vi "NEW数据采集传输系统.vi"() -> ()   [LabVIEW 2016, in "数据传输系统.lvlib"]
uses:
  <vilib>/Averna/Notify Icon/NotifyIcon.llb/BalloonIcon.ctl
  <vilib>/Utility/miscctls.llb/LVPointTypeDef.ctl
  <vilib>/Utility/config.llb/Read Key (String).vi
  <vilib>/Averna/Notify Icon/NotifyIcon.llb/GetSelectedItemEvent.vi
  <vilib>/Averna/Notify Icon/NotifyIcon.llb/SetVisible.vi
  <vilib>/Averna/Notify Icon/NotifyIcon.llb/SetMenuDefaultItem.vi
  <vilib>/Averna/Notify Icon/NotifyIcon.llb/SetTipText.vi
  <vilib>/Utility/config.llb/NI_LVConfig.lvlib
  data/FreeMem.dll
  <vilib>/Averna/Notify Icon/NotifyIcon.llb/NotifyIcon.lvclass
  <vilib>/ptbypt/NI_PtbyPt.lvlib
panel:
  in  "updateconfiguration":T1={"主机"="27.154.58.30", "用户"="update", "密码"="std23506", "远程路径"="数据传输系统\\平台数据传输系统.exe", "下载文件名"="平台数据传输系统.exe", "软件版本"=""}
  out "标题显示":string
  in  "更新":bool
  out "错误输出":errorcluster
  in  "停止输入":bool caption="停止 2"
  in  "系统编码选择框":string(combo)="地表水质量监测"
  in  "数据发送通道":enum16{"TCP", "VISA"}(ring)
  in  "baud rate":u32=9600 caption="波特率"
  in  "VISA resource name":refnum<visa-resource-name> caption="VISA资源名称"
  in  "实时数据发送时间间隔/min":i32=1
  in  "数据组合发送":bool
  in  "日志、参数发送":bool
  in  "2011发送":bool
  in  "判断数据反馈":bool
  in  "数据发送协议":enum16{"2005-212协议", "2017-212协议"}(ring)=enum."2017-212协议"
  in  "重发时间":T2(ring)
  in  "重发日期":T3(ring)
  in  "开机启动":bool
  in  "确定更改起始时间":bool
  in  "更改起始时间":bool
  in  "数据发送起始时间":timestamp format="%<%.3X\n%Y/%m/%d>T"
  in  "每周自动重发":bool=TRUE
  in  "确定":bool
  in  "返回":bool
  in  "PW":string
  in  "MN":string
  in  "PORT":string
  in  "IP":string
  in  "站点设备":string
  in  "站点名称":string
  out "设置超时时间/min":i32=1
  out "状态信息":T4={"1st Error to Convert "=63, "步骤 "=enum."发送数据", "元素"="实时数据", "TCP服务端掉线计数"=0, "TCP掉线时间节点"="2019/05/08 15:24:17"} {"1st Error to Convert" items=["无错误", "参数错误", "内存已满", "超出区域", "文件结束", "文件已打开", "一般文件IO错误", "未找到文件", "文件权限错误", "磁盘已满", "路径副本", "打开过多文件", "未启用", "未找到资源文件", "无法添加资源", "未找到资源", "未找到图像", "图像内存错误", "画笔不存在", "配置错误类型", "配置未找到解析段", "配置解析错误", "配置内存错误", "错误外部代码格式", "错误外部代码偏移量", "外部代码不存在", "空窗口", "销毁窗口错误", "空菜单", "打印已中止", "错误打印记录", "打印驱动程序错误", "打印时窗口错误", "打印时内存错误", "打印对话框错误", "一般打印错误", "无效设备引用句柄", "设备未找到", "设备参数错误", "设备单位错误", "无法打开设备", "设备调用已中止", "一般错误", "用户已取消", "对象ID过低", "对象ID过高", "对象不在堆中", "未知的堆", "错误DefProc ID", "DefProc不在表格中", "范围外信息", "空方法", "未知信息", "不支持管理器调用", "错误地址", "连接过程中", "连接超时", "连接过程中", "不支持网络属性", "网络错误", "正在使用的地址", "系统缺少内存", "连接已中止", "连接已拒绝", "连接未建立", "连接已建立", "连接已关闭", "初始化错误（交互应用程序管理器）", "错误事件发生", "等待无约束事件发生处理程序", "事件发生队列溢出", "错误路径", "未发出信号量", "未识别类型（交互应用程序管理器）"]}
  out "数据接收超时指示灯":bool
  out "空闲时间/s":string
  out "系统时间":string
  out "实时小时数据上传":bool
  out "系统状态改变":bool
  out "软件版本":string
  out "掉线指示":bool
  out "核查数据上传":bool
  out "配置信息":T5
  in  "参数配置":bool
  out "反控数据发送":bool
  out "读取报文显示":string
  out "发送报文显示":string
  out "心跳包":bool
  out "通信状态":bool
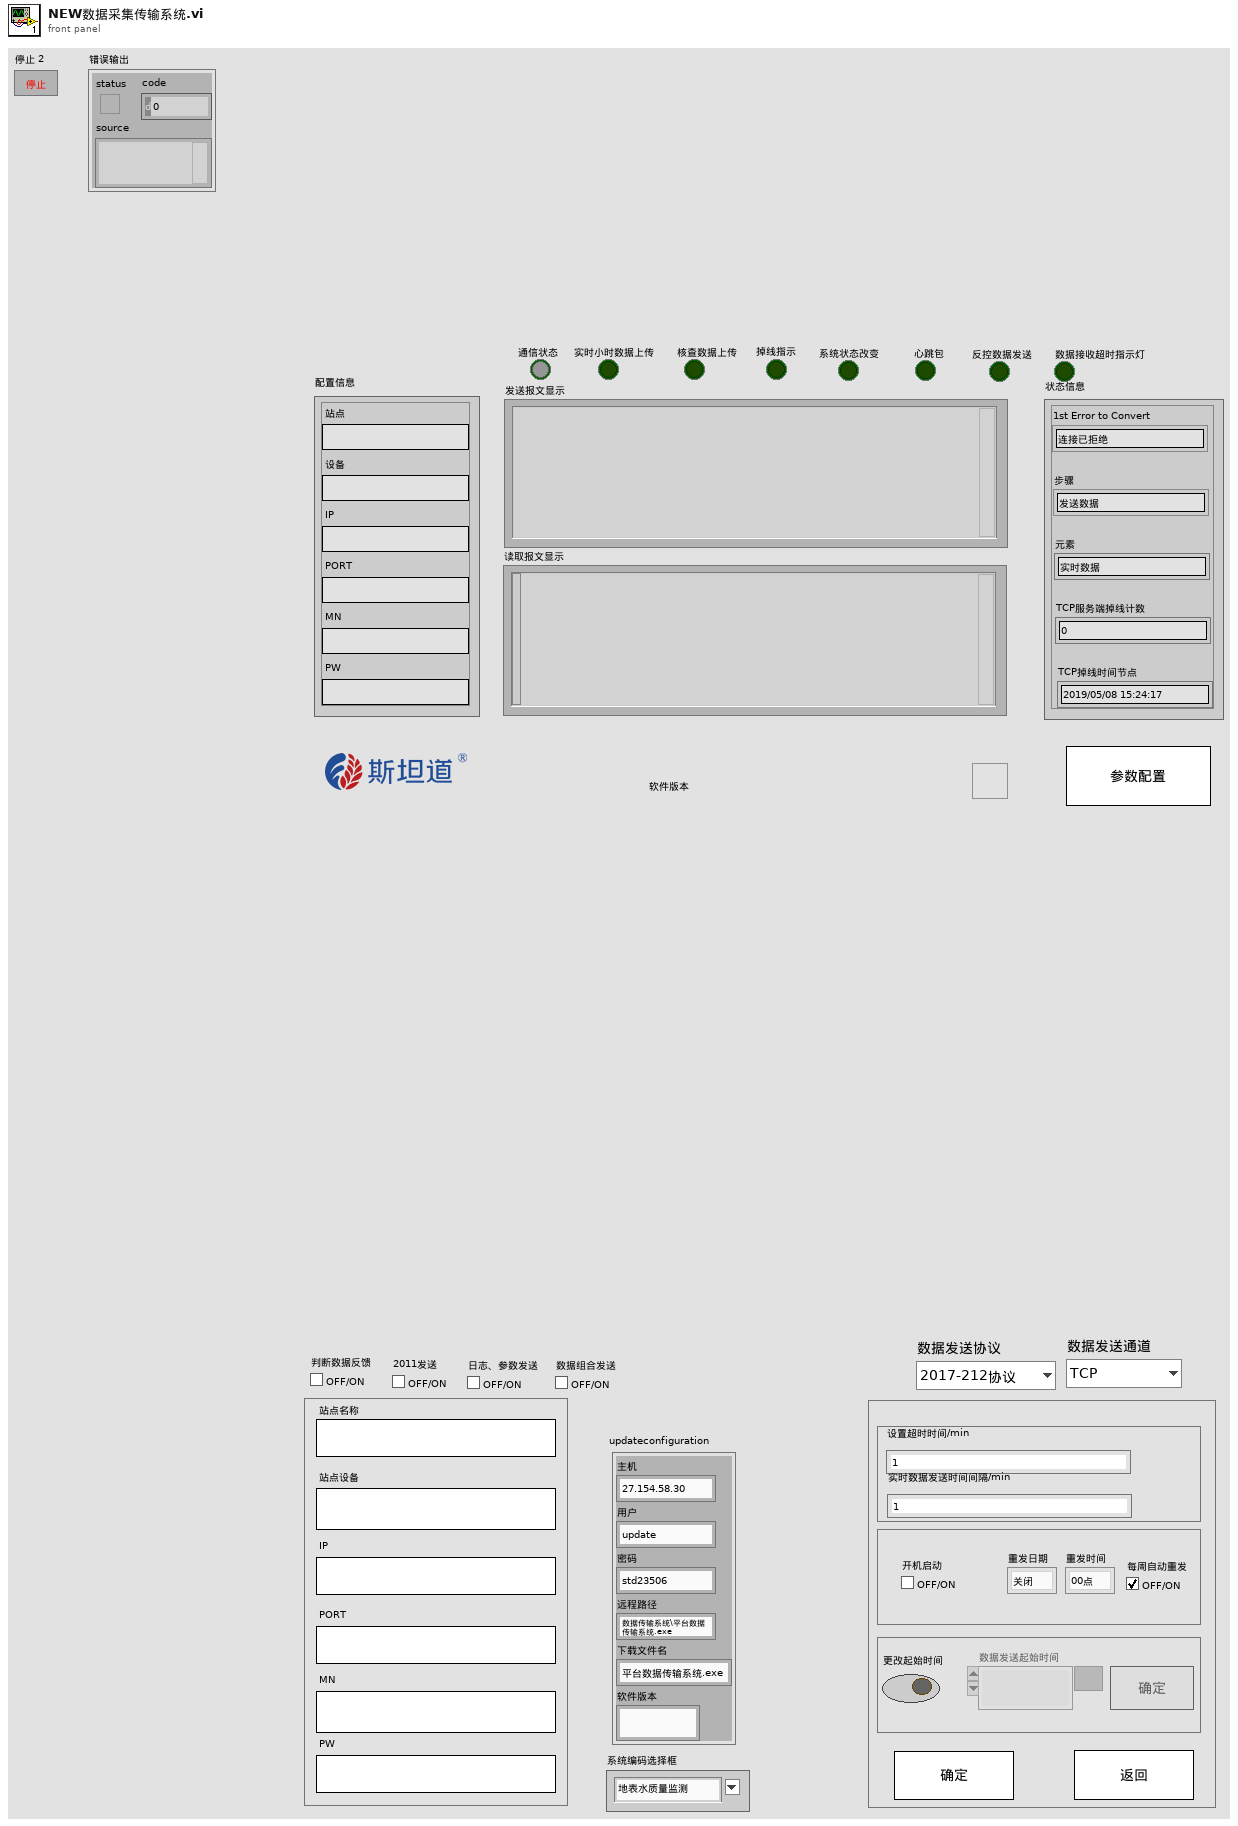
[diagram p1: front panel]
types:
  T1 = cluster{"主机":string, "用户":string, "密码":string, "远程路径":string, "下载文件名":string, "软件版本":string}
  T2 = enum16{"00点", "01点", "02点", "03点", "04点", "05点", "06点", "07点", "08点", "09点", "10点", "11点", "12点", "13点", "14点", "15点", "16点", "17点", "18点", "19点", "20点", "21点", "22点", "23点"}
  T3 = enum16{"关闭", "星期日", "星期一", "星期二", "星期三", "星期四", "星期五", "星期六"}
  T4 = cluster{"1st Error to Convert ":i32, "步骤 ":enum16{"打开连接", "发送数据", "读取数据", "数据处理", "关闭连接"}, "元素":string, "TCP服务端掉线计数":i32, "TCP掉线时间节点":string}
  T5 = cluster{"站点":string, "设备":string, "IP":string, "PORT":string, "MN":string, "PW":string}
  T6 = typedef "LVDateTimeRec.ctl" = cluster{"秒数的小数部分":dbl, "秒":i32, "分":i32, "时":i32, "日":i32, "月":i32, "年":i32, "天数（周）":i32, "天数（年）":i32, "DST":i32}
  T7 = enum32{"invalid app kind", "Development System", "Run Time System", "Student Edition", "Embedded LabVIEW", "Evaluation", "Custom"}
  T8 = typedef "LVPointTypeDef.ctl" = cluster{"Horizontal":i16, "Vertical":i16}
  T9 = cluster{"CODMn":bool, "CODCr":bool, "DO":bool, "铜":bool, "PH":bool, "氨氮":bool, "比电导率":bool, "水温":bool, "COD":bool, "浊度":bool, "总氮":bool, "总磷":bool, "叶绿素a":bool, "藻密度":bool, "水位":bool, "流速":bool, "瞬时流量":bool, "累积流量":bool, "亚硝酸盐":bool, "硫化物":bool, "ORP":bool, "铅":bool, "镉":bool, "锌":bool, "镍":bool, "锰":bool, "汞":bool}
  T10 = typedef "NI_LVConfig.lvlib/Config Data RefNum.ctl" = refnum<k1>
  T11 = typedef "imagedata.ctl" = cluster{"image type":i32, "image depth":i32, "image":u8[], "mask":u8[], "colors":u32[], "Rectangle":cluster{"left":i16, "top":i16, "right":i16, "bottom":i16}}
  T12 = cluster{"[0]":string, "[1]":string, "[2]":string, "[3]":string, "[4]":string, "[5]":string, "[6]":string, "[7]":string, "[8]":string, "[9]":string, "[10]":string, "[11]":string, "[12]":string, "[13]":string, "[14]":string, "[15]":string, "[16]":string, "[17]":string, "[18]":string, "[19]":string, "[20]":string, "[21]":string, "[22]":string, "[23]":string, "[24]":string, "[25]":string, "[26]":string}
  T13 = enum8{"Enabled", "Disabled", "Disabled and Grayed Out"}
  T14 = cluster{"[0]":string, "[1]":string, "[2]":string, "[3]":string, "[4]":string, "[5]":string, "[6]":string, "[7]":string}
  T15 = cluster{"[0]":string, "[1]":string, "[2]":string, "[3]":string, "[4]":string, "[5]":string, "[6]":string, "[7]":string, "[8]":string, "[9]":string, "[10]":string, "[11]":string, "[12]":string, "[13]":string, "[14]":string}
  T16 = enum32{"Invalid", "Standard", "Closed", "Hidden", "Minimized", "Maximized"}
  T17 = typedef "NotifyIcon.lvlib/NotifyIcon.lvclass/BalloonIcon.ctl" = enum32{"None", "Information", "Warning", "Error"}
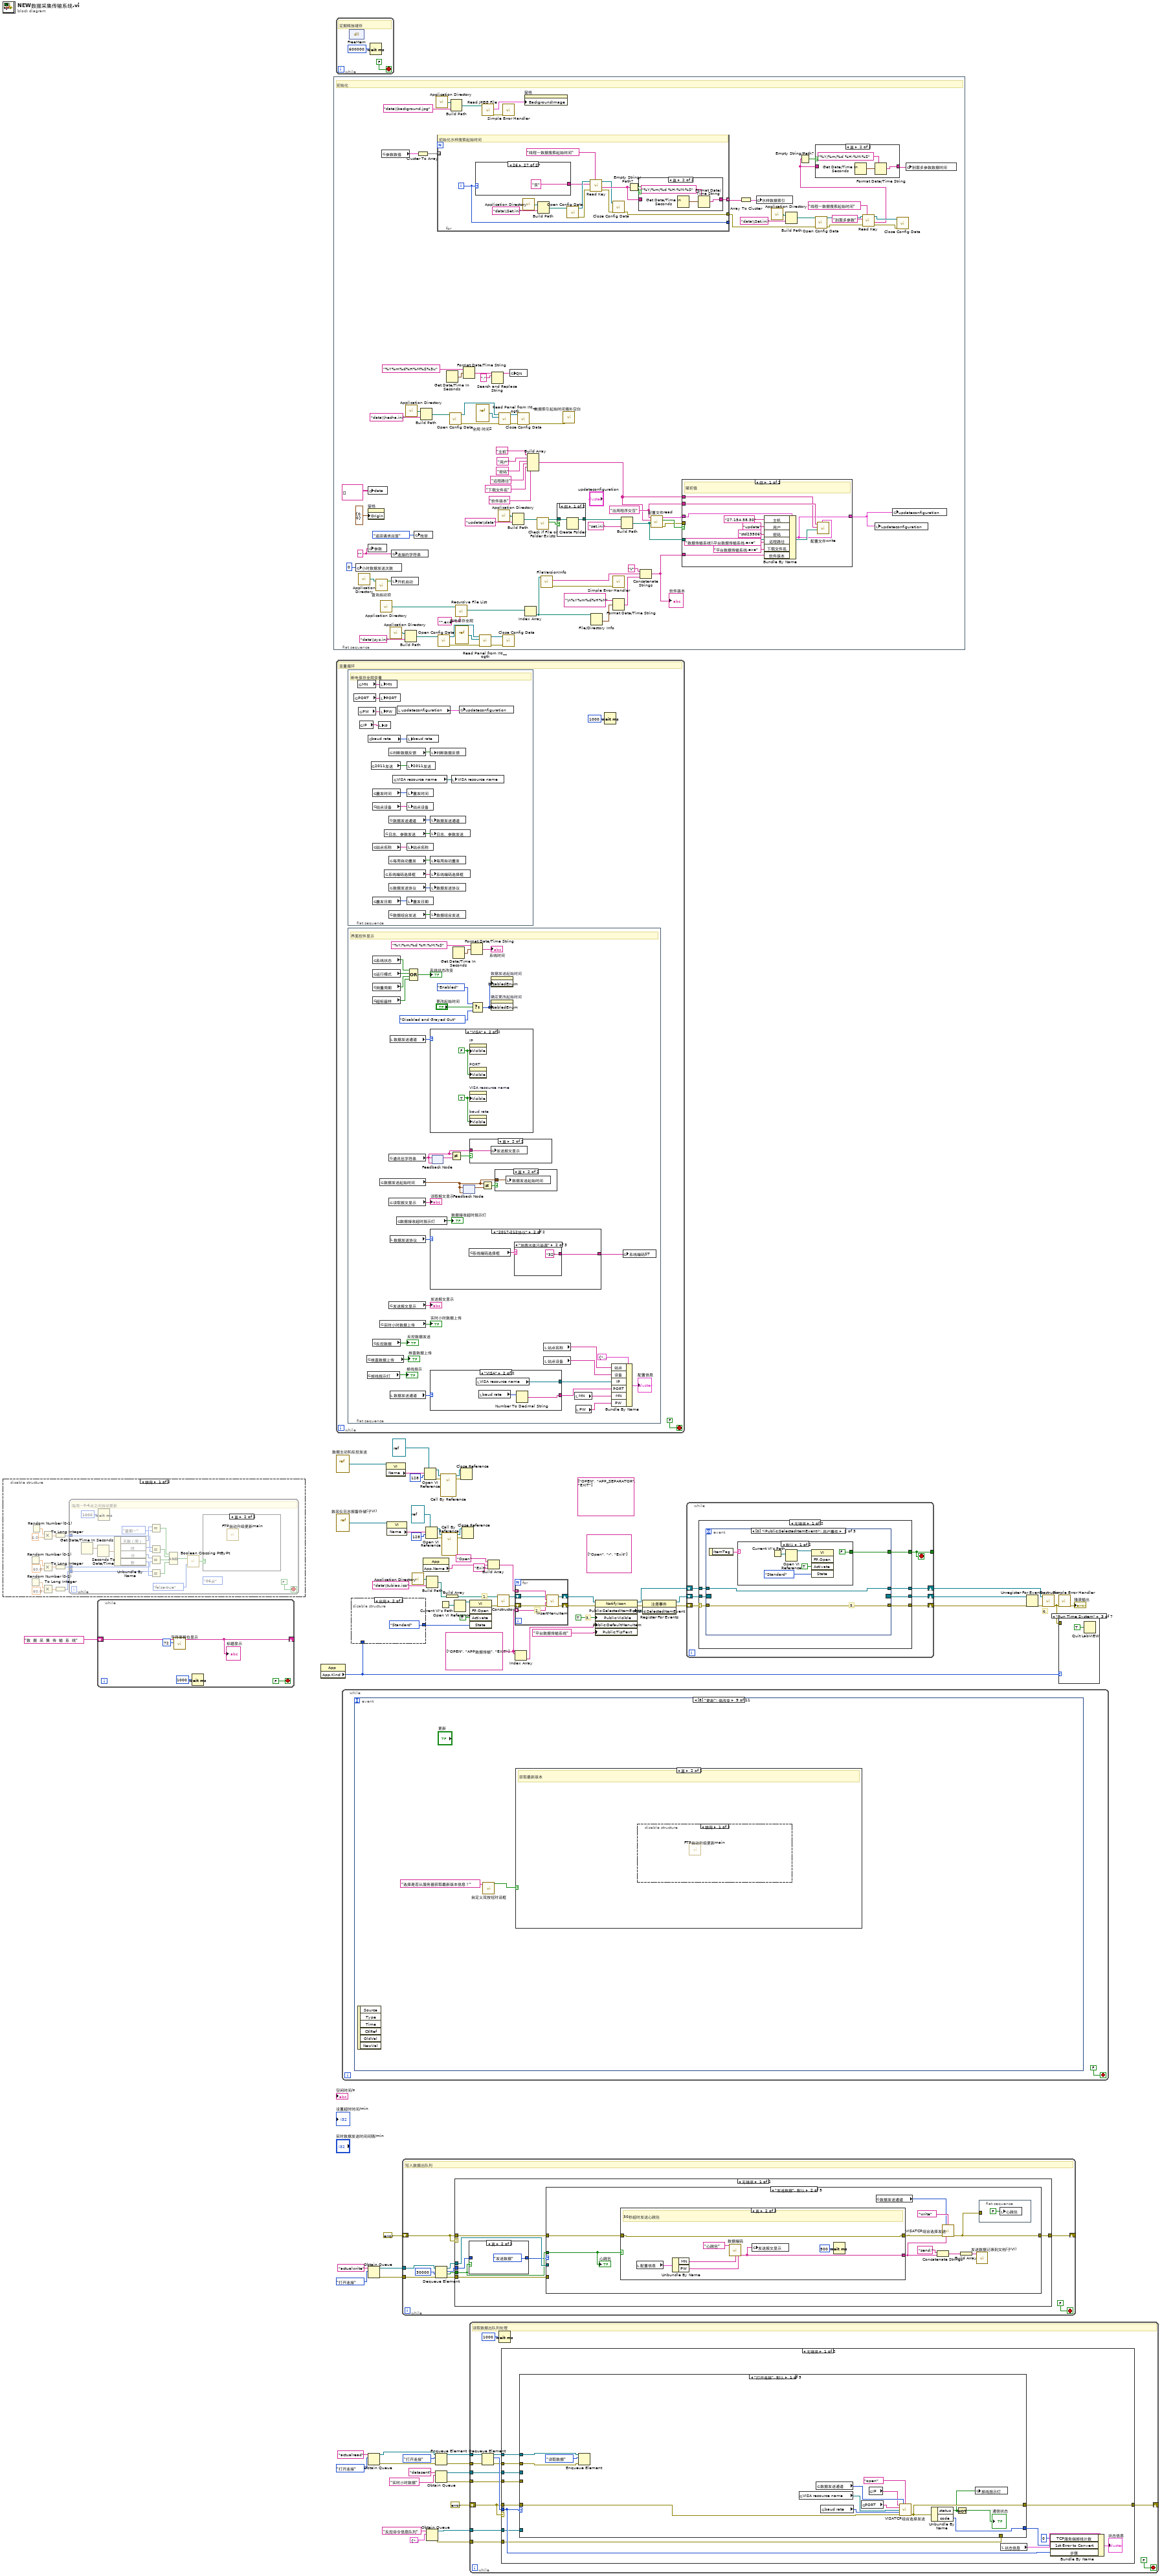
[diagram p0: block diagram]
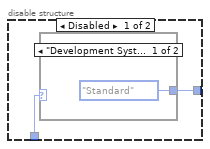
[diagram p4: hidden frame]
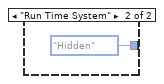
[diagram p5: hidden frame]
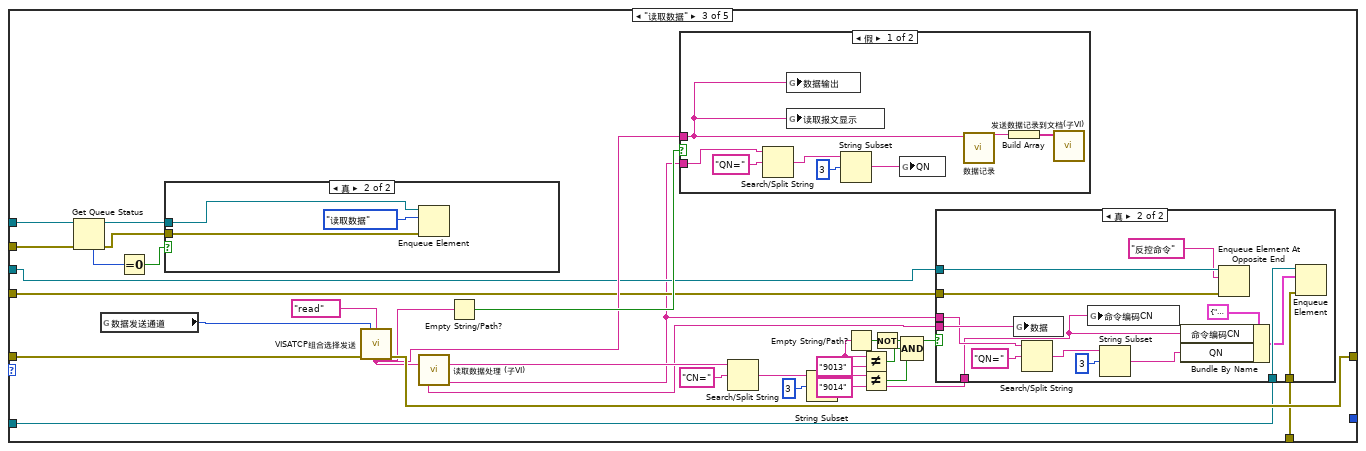
[diagram p7: hidden frame]
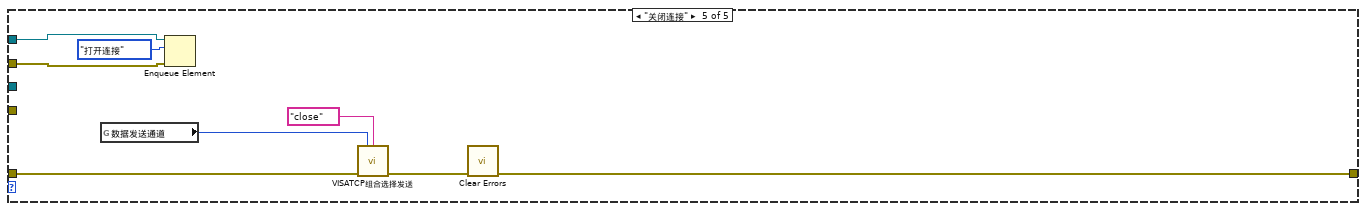
[diagram p12: hidden frame]
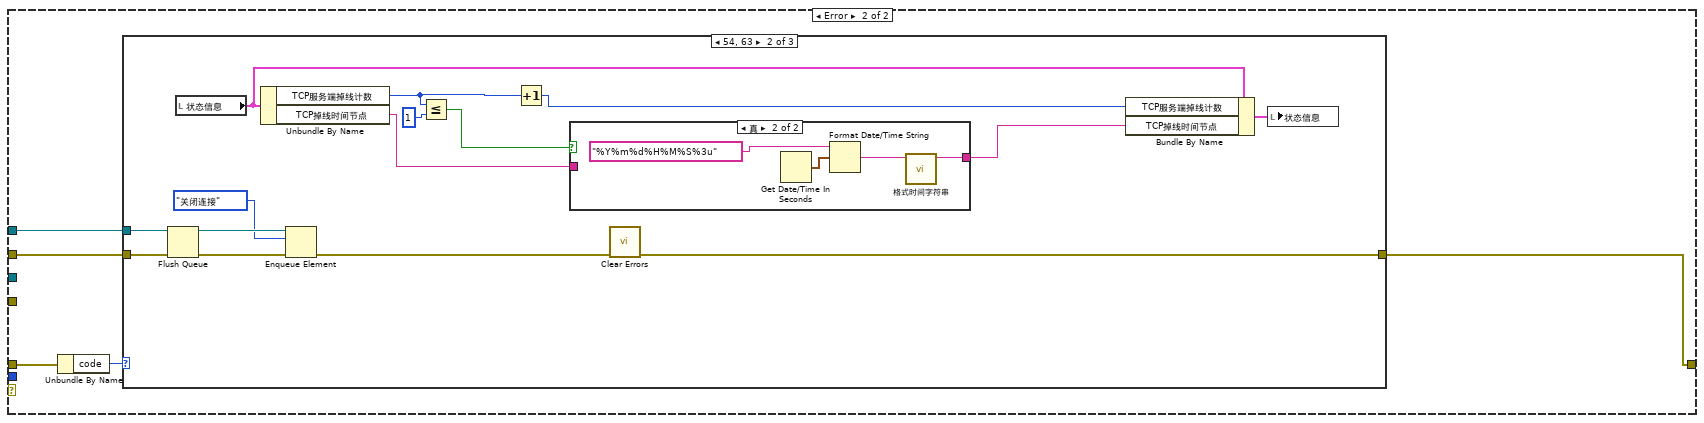
[diagram p13: hidden frame]
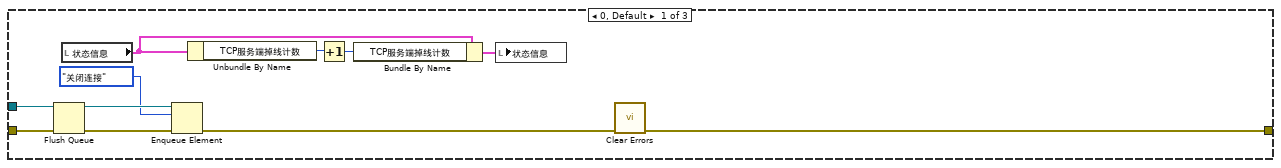
[diagram p14: hidden frame]
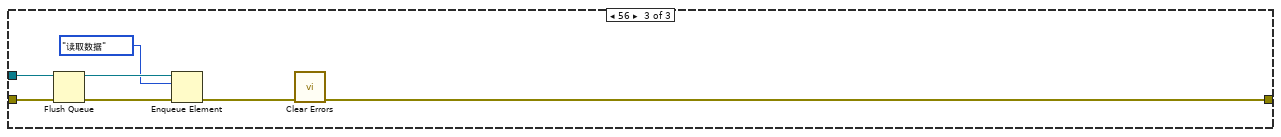
[diagram p16: hidden frame]
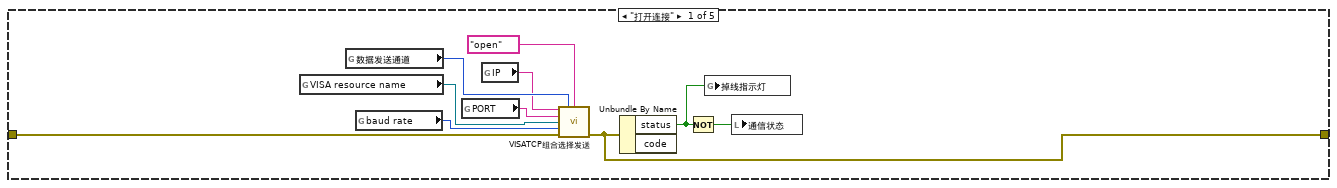
[diagram p18: hidden frame]
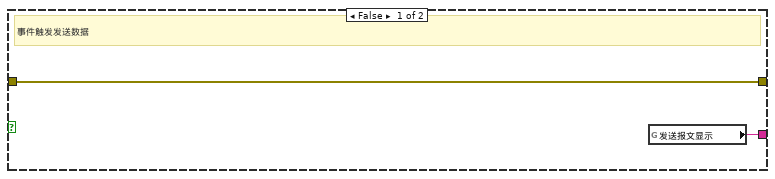
[diagram p19: hidden frame]
diagram:
  w1 = string[] ["OPEN", "APP数据传输", "EXIT"]
  (unwired) string[] ["OPEN", "APP_SEPARATOR", "EXIT"]
  (unwired) string[] ["Open", "-", "Exit"]
  # "6."
  # "3."
  # "1."
  n1 = disable-structure shown="禁用" {
    frame Disabled {
      n2 = Random Number (0-1)() -> (number: 0 to 1=w80:dbl)
      n3 = Random Number (0-1)() -> (number: 0 to 1=w79:dbl)
      n4 = Random Number (0-1)() -> (number: 0 to 1=w83:dbl)
      n5 = Multiply(x=w83, y=6.0) -> (x*y=w77:dbl)
      n6 = Multiply(x=w80, y=60.0) -> (x*y=w75:dbl)
      n7 = Multiply(x=w79, y=60.0) -> (x*y=w73:dbl)
      n8 = To Long Integer(number=w77) -> (32bit integer=w76:i32)
      n9 = To Long Integer(number=w75) -> (32bit integer=w74:i32)
      n10 = To Long Integer(number=w73) -> (32bit integer=w72:i32)
      n11 = while {
        tunnel: w76 -> [w91]
        tunnel: w74 -> [w86]
        tunnel: w72 -> [w85]
        stop <- FALSE stop-if-true
        (unwired) T2."06点" ("重发时间")
        # "每周一0-6点之间自动更新"
        n12 = Get Date/Time In Seconds() -> (seconds since 1Jan1904=w100:timestamp)
        n13 = Seconds To Date/Time(time stamp (now)=w100) -> (date time rec=w96:T6)  [unwired: 1 in]
        n14 = Wait (ms)(milliseconds to wait=u32 1000 ("等待时间（毫秒）")) -> ()  [unwired: 1 out]
        n15 = Unbundle By Name(w96) -> ("天数（周）"=w99:i32, "时"=w93:i32, "分"=w90:i32, "秒"=w88:i32)
        n16 = Equal?(x=w99, y=T3."星期一" ("重发日期")) -> (x = y?=w98:bool)
        n17 = Equal?(x=w93, y=w91) -> (x = y?=w97:bool)
        n18 = Equal?(x=w90, y=w86) -> (x = y?=w89:bool)
        n19 = Equal?(x=w85, y=w88) -> (x = y?=w87:bool)
        n20 = Compound Arithmetic op=AND ("复合运算")(w98, w97, w89, w87) -> (w95:bool)
        n21 = call <vilib>:"Boolean Crossing PtByPt.vi"("direction"=enum16{"either", "false-true", "true-false"}."false-true", "input"=w95) -> ("crossing"=w84:bool)  [unwired: 1 in]
        n22 = case shown="真" w84 {
          frame False {
          }
          frame True {
            n23 = call "FTP自动升级更新main.vi"() -> ()  [unwired: 12 in]
          }
        }
      }
    }
    frame Enabled {
    }
  }
  n24 = while {
    shift-right: [w104] -> _
    shift-left: "数  据  采  集  传  输  系  统" ("标题显示") -> [w105]
    stop <- FALSE stop-if-true
    n25 = call "字符串移位显示.vi"("字符框大小"=72, "字符串输入"=w105) -> ("移位后字符串"=w104:string)  [unwired: 8 in, 1 out]
    "标题显示" <- w104
    n26 = Wait (ms)(milliseconds to wait=u32 1000 ("等待时间（毫秒）")) -> ()  [unwired: 1 out]
  }
  n27 = property class="App"() -> ("App.Kind"=w46:T7)  [unwired: 2 in, 2 out]
  n28 = flat-sequence {
    frame #0 {
      w137 = "应用程序交互" ("section")
      w187 = "" ("参数")
      # "初始化"
      n29 = global write "全局 小时数据发送次数.vi" "小时数据发送次数"(0 ("数值")) -> ()
      n30 = call <vilib>:"Application Directory.vi"() -> ("Application Directory"=w157:path)
      n31 = global write "全局 实时数据参数.vi" "data"(string[][] [] ("data")) -> ()
      n32 = property on="窗格" class="Pane"("Origin"=T8 {"Horizontal"=0, "Vertical"=0} ("原点")) -> ()  [unwired: 2 in, 2 out]
      n33 = global write "全局 实时数据参数.vi" "参数"(w187) -> ()
      n34 = call "查询启动项.vi"("启动文件路径"=w157) -> ("包含启动项"=w156:bool)  [unwired: 9 in, 1 out]
      n35 = call <vilib>:"Application Directory.vi"() -> ("Application Directory"=w167:path)
      n36 = global read "全局1.vi" "参数数值"() -> (w143:T9)
      n37 = call <vilib>:"Application Directory.vi"() -> ("Application Directory"=w161:path)
      n38 = global write "全局 实时数据参数.vi" "连接的字符串"(w187) -> ()
      n39 = local write "开机启动"(w156) -> ()
      n40 = Build Path(base path=w161, name or relative path="data\\sys.ini" ("名称或相对路径")) -> (appended path=w159:path)
      n41 = call <vilib>:"Application Directory.vi"() -> ("Application Directory"=w151:path)
      n42 = global write "全局1.vi" "枚举"(enum16{"返回请求应答", "上传数据", "返回执行结果"}."返回请求应答" ("枚举")) -> ()
      n43 = Cluster To Array(cluster=w143) -> (array=w144:bool[])
      n44 = Build Path(base path=w151, name or relative path="data\\hecha.ini" ("名称或相对路径")) -> (appended path=w153:path)
      n45 = call <vilib>:"Application Directory.vi"() -> ("Application Directory"=w178:path)
      n46 = for {
        tunnel: w144 -> [_] mode=indexing
        tunnel: [w219] -> _
        tunnel: [w216] -> w142 mode=indexing
        tunnel: [w215] -> w117
        i -> [w219]
        # "初始化水样搜索起始时间"
        n47 = case shown="26" w219 {
          tunnel: ["CODMn" "CODCr" "DO" "铜" "PH" "氨氮" "比电导率" "水温" "COD" "浊度" "总氮" "总磷" "叶绿素a" "藻密度" "水位" "流速" "瞬时流量" "累积流量" "亚硝氮" "硫化物" "ORP" "铅" "镉" "锌" "镍" "锰" "汞"] -> w222
          frame 0, Default {
          }
          frame 1 {
          }
          frame 2 {
          }
          frame 3 {
          }
          frame 4 {
          }
          frame 5 {
          }
          frame 6 {
          }
          frame 7 {
          }
          frame 8 {
          }
          frame 9 {
          }
          frame 10 {
          }
          frame 11 {
          }
          frame 12 {
          }
          frame 13 {
          }
          frame 14 {
          }
          frame 15 {
          }
          frame 16 {
          }
          frame 17 {
          }
          frame 18 {
          }
          frame 19 {
          }
          frame 20 {
          }
          frame 21 {
          }
          frame 22 {
          }
          frame 23 {
          }
          frame 24 {
          }
          frame 25 {
          }
          frame 26 {
          }
        }
        n48 = call <vilib>:"Application Directory.vi"() -> ("Application Directory"=w228:path)
        n49 = Build Path(base path=w228, name or relative path="data\\Set.ini" ("名称或相对路径")) -> (appended path=w226:path)
        n50 = call <vilib>:"Open Config Data.vi"("configuration file path"=w226) -> ("error out"=w224:errorcluster, "refnum"=w225:T10)  [unwired: 8 in, 1 out]
        n51 = call-poly <vilib>:"Read Key.vi"("section"="线程一数据搜索起始时间", "error in (no error)"=w224, "key"=w222, "refnum"=w225) -> ("error out"=w217:errorcluster, "value"=w220:string, "refnum out"=w218:T10)  [unwired: 4 in, 1 out]
        n52 = call <vilib>:"Close Config Data.vi"("error in (no error)"=w217, "refnum"=w218) -> ("error out"=w215:errorcluster)  [unwired: 8 in, 1 out]
        n53 = Empty String/Path?(string/path=w220) -> (empty?=w221:bool)
        n54 = case shown="真" w221 {
          tunnel: [w229 w230] -> w216
          tunnel: w220 -> [w229 _]
          frame False {
          }
          frame True {
            n55 = Get Date/Time In Seconds() -> (seconds since 1Jan1904=w232:timestamp)
            n56 = Format Date/Time String(time format string (%c)="%Y/%m/%d %H:%M:%S" ("时间格式字符串(%c)"), seconds (now)=w232) -> (date/time string=w230:string)  [unwired: 1 in]
          }
        }
      }
      n57 = call <vilib>:"Open Config Data.vi"("configuration file path"=w159) -> ("error out"=w165:errorcluster, "refnum"=w164:T10)  [unwired: 8 in, 1 out]
      n58 = Get Date/Time In Seconds() -> (seconds since 1Jan1904=w183:timestamp)
      n59 = call <vilib>:"Open Config Data.vi"("configuration file path"=w153) -> ("error out"=w147:errorcluster, "refnum"=w148:T10)  [unwired: 8 in, 1 out]
      n60 = Build Path(base path=w178, name or relative path="data\\background.jpg" ("名称或相对路径")) -> (appended path=w177:path)
      n61 = call <vilib>:"Recursive File List.vi"("pattern"="*.exe", "Folder Path"=w167) -> ("All Files in Dir"=w173:path[])  [unwired: 5 in, 4 out]
      n62 = vi-ref "断电保存全局.vi"() -> (w163:refnum<vi>)
      n63 = Format Date/Time String(time format string (%c)="%Y%m%d%H%M%S%3u" ("时间格式字符串(%c)"), seconds (now)=w183) -> (date/time string=w182:string)  [unwired: 1 in]
      n64 = vi-ref "全局 时间2.vi"() -> (w149:refnum<vi>)
      n65 = call <userlib>:"Read Panel from INI__ogtk.vi"("error in (no error)"=w165, "VI ref"=w163, "refnum"=w164) -> ("error out"=w158:errorcluster, "refnum out"=w162:T10)  [unwired: 7 in]
      n66 = call <vilib>:"Read JPEG File.vi"("path to JPEG file"=w177) -> ("error out"=w175:errorcluster, "image data"=w176:T11)  [unwired: 8 in, 1 out]
      n67 = Search and Replace String(input string=w182, search string="." ("搜索字符串")) -> (result string=w180:string)  [unwired: 6 in, 3 out]
      n68 = call <vilib>:"Application Directory.vi"() -> ("Application Directory"=w123:path)
      n69 = call <userlib>:"Read Panel from INI__ogtk.vi"("error in (no error)"=w147, "VI ref"=w149, "refnum"=w148) -> ("error out"=w146:errorcluster, "refnum out"=w150:T10)  [unwired: 7 in]
      n70 = call <vilib>:"Simple Error Handler.vi"("error in (no error)"=w175) -> ()  [unwired: 4 in, 5 out]
      n71 = call <vilib>:"Close Config Data.vi"("error in (no error)"=w158, "refnum"=w162) -> ()  [unwired: 8 in, 2 out]
      n72 = global write "全局1.vi" "QN"(w180) -> ()
      n73 = Build Path(base path=w123, name or relative path="update\\data" ("名称或相对路径")) -> (appended path=w124:path)
      n74 = call <vilib>:"Close Config Data.vi"("error in (no error)"=w146, "refnum"=w150) -> ("error out"=w145:errorcluster)  [unwired: 8 in, 1 out]
      n75 = property on="窗格" class="Pane"("BackgroundImage"=w176) -> ()  [unwired: 2 in, 2 out]
      n76 = Index Array(array=w173) -> (element=w172:path)  [unwired: 1 in]
      n77 = Build Array("主机" ("section"), "用户" ("section"), "密码" ("key"), "远程路径" ("key"), "下载文件名" ("key"), "软件版本" ("key")) -> (w127:string[])
      n78 = call <vilib>:"Check if File or Folder Exists.vi"("path"=w124) -> ("file or folder exists?"=w125:bool, "dup path"=w126:path)  [unwired: 8 in, 1 out]
      n79 = call <vilib>:"FileVersionInfo.vi"("Application Path in"=w172) -> ("error out"=w166:errorcluster, "File Version Info"=w154:string)  [unwired: 7 in, 2 out]
      n80 = case shown="假" w125 {
        tunnel: w126 -> [w195 w196]
        tunnel: [w194 w196] -> w121
        frame False {
          n81 = Create Folder(path (use dialog)=w195) -> (created path=w194:path)  [unwired: 2 in, 2 out]
        }
        frame True {
        }
      }
      n82 = call "数据索引起始时间填补空白.vi"("error in (no error)"=w145) -> ()  [unwired: 10 in, 1 out]
      n83 = File/Directory Info(path=w172) -> (last mod=w171:timestamp)  [unwired: 1 in, 6 out]
      n84 = call <vilib>:"Simple Error Handler.vi"("error in (no error)"=w166) -> ()  [unwired: 4 in, 5 out]
      n85 = Format Date/Time String(time format string (%c)="\n%Y%m%d%H%M" ("时间格式字符串(%c)"), seconds (now)=w171) -> (date/time string=w168:string)  [unwired: 1 in]
      n86 = Build Path(base path=w121, name or relative path="set.ini" ("名称或相对路径")) -> (appended path=w136:path)
      n87 = Concatenate Strings("V" ("字符串"), w154, w168) -> (w138:string)
      "软件版本" <- w138
      n88 = call "配置文件read.vi"("configuration file path"=w136, "键数组"=w127, "段"=w137) -> ("error out"=w135:errorcluster, "section exists?"=w140:bool, "updateconfiguration"=w139:T1)  [unwired: 6 in]
      n89 = case shown="假" w140 {
        tunnel: w139 -> [w203 w209]
        tunnel: [w202 w208] -> w134
        tunnel: w138 -> [w197 w214]
        tunnel: w137 -> [w206 w213]
        tunnel: w127 -> [w205 w212]
        tunnel: w136 -> [w204 w211]
        tunnel: w135 -> [_ w210]
        frame False {
          # "赋初值"
          n90 = Bundle By Name(cluster=w203, "主机"="27.154.58.30" ("key"), "用户"="update", "密码"="std23506", "远程路径"="数据传输系统\\平台数据传输系统.exe", "下载文件名"="平台数据传输系统.exe", "软件版本"=w197) -> (w202:T1)
          n91 = call "配置文件write.vi"("updateconfiguration"=w202, "configuration file path"=w204, "键数组"=w205, "段"=w206) -> ()  [unwired: 7 in, 1 out]
        }
        frame True {
          # "本地"
          n92 = Bundle By Name(cluster=w209, "软件版本"=w214) -> (w208:T1)
          n93 = call "配置文件write.vi"("updateconfiguration"=w208, "error in (no error)"=w210, "configuration file path"=w211, "键数组"=w212, "段"=w213) -> ()  [unwired: 6 in, 1 out]
        }
      }
      n94 = Array To Cluster(array=w142) -> (cluster=w141:T12)
      n95 = global write "全局 水样时间.vi" "水样数据索引"(w141) -> ()
      n96 = call <vilib>:"Application Directory.vi"() -> ("Application Directory"=w120:path)
      n97 = Build Path(base path=w120, name or relative path="data\\Set.ini" ("名称或相对路径")) -> (appended path=w118:path)
      n98 = call <vilib>:"Open Config Data.vi"("error in (no error)"=w117, "configuration file path"=w118) -> ("error out"=w114:errorcluster, "refnum"=w115:T10)  [unwired: 7 in, 1 out]
      n99 = call-poly <vilib>:"Read Key.vi"("section"="线程一数据搜索起始时间", "error in (no error)"=w114, "key"="剖面多参数", "refnum"=w115) -> ("error out"=w111:errorcluster, "value"=w109:string, "refnum out"=w112:T10)  [unwired: 4 in, 1 out]
      n100 = Empty String/Path?(string/path=w109) -> (empty?=w108:bool)
      n101 = case shown="真" w108 {
        tunnel: [w190 w191] -> w110
        tunnel: w109 -> [w190 _]
        frame False {
        }
        frame True {
          n102 = Get Date/Time In Seconds() -> (seconds since 1Jan1904=w193:timestamp)
          n103 = Format Date/Time String(time format string (%c)="%Y/%m/%d %H:%M:%S" ("时间格式字符串(%c)"), seconds (now)=w193) -> (date/time string=w191:string)  [unwired: 1 in]
        }
      }
      n104 = local write "updateconfiguration"(w134) -> ()
      n105 = global write "update全局.vi" "updateconfiguration"(w134) -> ()
      n106 = call <vilib>:"Close Config Data.vi"("error in (no error)"=w111, "refnum"=w112) -> ()  [unwired: 8 in, 2 out]
      n107 = global write "全局 水样时间.vi" "剖面多参数数据时间"(w110) -> ()
    }
  }
  n108 = while {
    stop <- FALSE stop-if-true
    # "定期释放缓存"
    n109 = dll-call lib="PTH2fabs F\tgitkrakenCC;平台数采程序 - V2（微站认证版） - 整点触发dataFreeMem.dll" fn="FreeMem"() -> ()  [unwired: 4 in, 2 out]
    n110 = Wait (ms)(milliseconds to wait=u32 600000 ("等待时间（毫秒）")) -> ()  [unwired: 1 out]
  }
  n111 = while {
    stop <- FALSE stop-if-true
    # "变量循环"
    n112 = flat-sequence {
      frame #0 {
        # "断电保存全局变量"
        n113 = global read "断电保存全局.vi" "PORT"() -> (w333:string)
        n114 = global read "断电保存全局.vi" "MN"() -> (w332:string)
        n115 = global read "断电保存全局.vi" "PW"() -> (w331:string)
        n116 = global read "断电保存全局.vi" "IP"() -> (w334:string)
        n117 = global read "断电保存全局.vi" "baud rate"() -> (w329:u32)
        n118 = global read "断电保存全局.vi" "2011发送"() -> (w325:bool)
        n119 = global read "断电保存全局.vi" "重发时间"() -> (w319:T2)
        n120 = global read "断电保存全局.vi" "站点设备"() -> (w335:string)
        n121 = global read "断电保存全局.vi" "站点名称"() -> (w336:string)
        n122 = global read "断电保存全局.vi" "重发日期"() -> (w327:T3)
        n123 = local write "IP"(w334) -> ()
        n124 = local write "MN"(w332) -> ()
        n125 = local write "PORT"(w333) -> ()
        n126 = local write "PW"(w331) -> ()
        n127 = global read "断电保存全局.vi" "日志、参数发送"() -> (w324:bool)
        n128 = global read "断电保存全局.vi" "系统编码选择框"() -> (w320:string)
        n129 = global read "断电保存全局.vi" "判断数据反馈"() -> (w326:bool)
        n130 = global read "断电保存全局.vi" "数据发送通道"() -> (w321:enum16{"TCP", "VISA"})
        n131 = global read "断电保存全局.vi" "每周自动重发"() -> (w328:bool)
        n132 = global read "断电保存全局.vi" "数据发送协议"() -> (w322:enum16{"2005-212协议", "2017-212协议"})
        n133 = global read "断电保存全局.vi" "数据组合发送"() -> (w323:bool)
        n134 = global read "断电保存全局.vi" "VISA resource name"() -> (w330:refnum<visa-resource-name>)
        n135 = local read "updateconfiguration"() -> (w318:T1)
        n136 = local write "baud rate"(w329) -> ()
        n137 = local write "2011发送"(w325) -> ()
        n138 = local write "重发时间"(w319) -> ()
        n139 = local write "站点设备"(w335) -> ()
        n140 = local write "站点名称"(w336) -> ()
        n141 = local write "重发日期"(w327) -> ()
        n142 = local write "判断数据反馈"(w326) -> ()
        n143 = local write "数据发送通道"(w321) -> ()
        n144 = local write "日志、参数发送"(w324) -> ()
        n145 = local write "每周自动重发"(w328) -> ()
        n146 = local write "系统编码选择框"(w320) -> ()
        n147 = local write "数据发送协议"(w322) -> ()
        n148 = local write "数据组合发送"(w323) -> ()
        n149 = local write "VISA resource name"(w330) -> ()
        n150 = global write "update全局.vi" "updateconfiguration"(w318) -> ()
      }
    }
    n151 = flat-sequence {
      frame #0 {
        # "界面控件显示"
        n152 = global read "全局1.vi" "核查数据上传"() -> (→"核查数据上传":bool)
        n153 = global read "全局 数据发送重叠.vi" "掉线指示灯"() -> (→"掉线指示":bool)
        n154 = global read "全局1.vi" "系统状态"() -> (w267:bool)
        n155 = global read "全局1.vi" "运行模式"() -> (w268:bool)
        n156 = global read "全局1.vi" "测量周期"() -> (w269:bool)
        n157 = global read "全局1.vi" "超标留样"() -> (w270:bool)
        n158 = global read "全局1.vi" "反控数据"() -> (→"反控数据发送":bool)
        n159 = global read "全局1.vi" "数据发送起始时间"() -> (w264:timestamp)
        n160 = global read "全局1.vi" "实时小时数据上传"() -> (→"实时小时数据上传":bool)
        n161 = global read "全局1.vi" "通讯包字符串"() -> (w281:string)
        n162 = global read "全局1.vi" "读取报文显示"() -> (→"读取报文显示":string)
        n163 = global read "全局1.vi" "发送报文显示"() -> (→"发送报文显示":string)
        n164 = local read "数据发送通道"() -> (w275:enum16{"TCP", "VISA"})
        n165 = local read "数据发送协议"() -> (w289:enum16{"2005-212协议", "2017-212协议"})
        n166 = local read "数据发送通道"() -> (w300:enum16{"TCP", "VISA"})
        n167 = global read "全局 数据发送重叠.vi" "数据接收超时指示灯"() -> (→"数据接收超时指示灯":bool)
        n168 = Compound Arithmetic op=OR ("复合运算")(w267, w268, w269, w270) -> (→"系统状态改变":bool)
        n169 = case shown="\"VISA\"" w275 {
          frame "TCP", Default {
            w302 = TRUE ("可见")
            w303 = FALSE ("可见")
            n170 = property on="IP" class="Str"("Visible"=w302) -> ()  [unwired: 2 in, 2 out]
            n171 = property on="PORT" class="Str"("Visible"=w302) -> ()  [unwired: 2 in, 2 out]
            n172 = property on="VISA resource name" class="VISAName"("Visible"=w303) -> ()  [unwired: 2 in, 2 out]
            n173 = property on="baud rate" class="DigNum (严格)"("Visible"=w303) -> ()  [unwired: 2 in, 2 out]
          }
          frame "VISA" {
            w304 = FALSE ("可见")
            w305 = TRUE ("可见")
            n174 = property on="IP" class="Str"("Visible"=w304) -> ()  [unwired: 2 in, 2 out]
            n175 = property on="PORT" class="Str"("Visible"=w304) -> ()  [unwired: 2 in, 2 out]
            n176 = property on="VISA resource name" class="VISAName"("Visible"=w305) -> ()  [unwired: 2 in, 2 out]
            n177 = property on="baud rate" class="DigNum (严格)"("Visible"=w305) -> ()  [unwired: 2 in, 2 out]
          }
        }
        n178 = case shown="\"2017-212协议\"" w289 {
          tunnel: ["32" ("设备编码MN") w308] -> w288
          frame "2005-212协议", Default {
          }
          frame "2017-212协议" {
            n179 = global read "断电保存全局.vi" "系统编码选择框"() -> (w309:string)
            n180 = case shown="\"地表水体污染源\"" w309 {
              tunnel: ["52" ("设备编码MN") "32" ("设备编码MN") "21" ("设备编码MN")] -> w308
              frame "污水排放过程监测" {
              }
              frame "地表水体污染源" {
              }
              frame "地表水质量监测", Default {
              }
            }
          }
        }
        n181 = case shown="\"VISA\"" w300 {
          tunnel: [w314 w317] -> w297
          tunnel: [w313 w315] -> w294
          frame "TCP", Default {
            n182 = local read "PORT"() -> (w313:string)
            n183 = local read "IP"() -> (w314:string)
          }
          frame "VISA" {
            n184 = local read "VISA resource name"() -> (w317:refnum<visa-resource-name>)
            n185 = local read "baud rate"() -> (w316:u32)
            n186 = Number To Decimal String(number=w316) -> (decimal integer string=w315:string)  [unwired: 1 in]
          }
        }
        n187 = feedback #1(w281) -> (w282:string)
        n188 = feedback-in #1(w281) -> ()
        n189 = Not Equal?(x=w281, y=w282) -> (x != y?=w280:bool)
        n190 = Get Date/Time In Seconds() -> (seconds since 1Jan1904=w290:timestamp)
        n191 = feedback #2(w264) -> (w266:timestamp)
        n192 = feedback-in #2(w264) -> ()
        n193 = case shown="真" w280 {
          tunnel: w281 -> [_ w306]
          frame False {
          }
          frame True {
            n194 = global write "全局1.vi" "发送报文显示"(w306) -> ()
          }
        }
        n195 = Format Date/Time String(time format string (%c)="%Y/%m/%d %H:%M:%S" ("时间格式字符串(%c)"), seconds (now)=w290) -> (date/time string=→"系统时间":string)  [unwired: 1 in]
        n196 = Select(t=T13."Enabled" ("禁用"), s="更改起始时间", f=T13."Disabled and Grayed Out" ("禁用")) -> (s? t:f=w276:T13)
        n197 = Not Equal?(x=w264, y=w266) -> (x != y?=w265:bool)
        n198 = property on="数据发送起始时间" class="AbsTime (严格)"("DisabledEnum"=w276) -> ()  [unwired: 2 in, 2 out]
        n199 = property on="确定更改起始时间" class="Bool"("DisabledEnum"=w276) -> ()  [unwired: 2 in, 2 out]
        n200 = case shown="真" w265 {
          tunnel: w264 -> [_ w301]
          frame False {
          }
          frame True {
            n201 = local write "数据发送起始时间"(w301) -> ()
          }
        }
        n202 = local read "站点名称"() -> (w296:string)
        n203 = local read "站点设备"() -> (w295:string)
        n204 = local read "MN"() -> (w293:string)
        n205 = local read "PW"() -> (w292:string)
        n206 = Bundle By Name(cluster=T5 {"站点"="", "设备"="", "IP"="", "PORT"="", "MN"="", "PW"=""} ("配置信息"), "站点"=w296, "设备"=w295, "IP"=w297, "PORT"=w294, "MN"=w293, "PW"=w292) -> (→"配置信息":T5)
        n207 = global write "全局1.vi" "系统编码ST"(w288) -> ()
      }
    }
    n208 = Wait (ms)(milliseconds to wait=u32 1000 ("等待时间（毫秒）")) -> ()  [unwired: 1 out]
  }
  n209 = vi-ref "数据主动和反控发送.vi"() -> (w37:refnum<vi>)
  n210 = vi-ref "数采仪日志报警存储(子VI).vi"() -> (w38:refnum<vi>)
  n211 = while {
    stop <- FALSE stop-if-true
    n212 = event shown="[8] \"更新\": 值改变" {
      selector: _ -> [_ _ _ _ _ _ _ _ _ _ _]
      dyn-events: _ -> [_ _ _ _ _ _ _ _ _ _ _]
      timeout: _ -> [_ _ _ _ _ _ _ _ _ _ _]
      event Timeout {
        n213 = event-data() -> ()  [unwired: 1 in, 3 out]
      }
      event "站点名称", "站点设备", "IP", "PORT", "MN", "PW", "VISA resource name", "baud rate", "系统编码选择框", "每周自动重发", "重发日期", "重发时间": Value Change {
        n214 = event-data() -> ()  [unwired: 1 in, 6 out]
        n215 = flat-sequence {
          frame #0 {
            n216 = global write "断电保存全局.vi" "PW"("PW") -> ()
            n217 = global write "断电保存全局.vi" "站点名称"("站点名称") -> ()
            n218 = global write "断电保存全局.vi" "MN"("MN") -> ()
            n219 = global write "断电保存全局.vi" "PORT"("PORT") -> ()
            n220 = global write "断电保存全局.vi" "IP"("IP") -> ()
            n221 = global write "断电保存全局.vi" "重发日期"("重发日期") -> ()
            n222 = global write "断电保存全局.vi" "重发时间"("重发时间") -> ()
            n223 = global write "断电保存全局.vi" "站点设备"("站点设备") -> ()
            n224 = global write "断电保存全局.vi" "baud rate"("baud rate") -> ()
            n225 = global write "断电保存全局.vi" "系统编码选择框"("系统编码选择框") -> ()
            n226 = global write "断电保存全局.vi" "每周自动重发"("每周自动重发") -> ()
            n227 = global write "断电保存全局.vi" "VISA resource name"("VISA resource name") -> ()
          }
          frame #1 {
            n228 = call <vilib>:"Application Directory.vi"() -> ("Application Directory"=w350:path)
            n229 = Build Path(base path=w350, name or relative path="data\\sys.ini" ("名称或相对路径")) -> (appended path=w352:path)
            n230 = call <vilib>:"Open Config Data.vi"("configuration file path"=w352) -> ("error out"=w356:errorcluster, "refnum"=w353:T10)  [unwired: 8 in, 1 out]
            n231 = vi-ref "断电保存全局.vi"() -> (w354:refnum<vi>)
            n232 = call <userlib>:"Write Panel to INI__ogtk.vi"("error in (no error)"=w356, "VI ref"=w354, "refnum"=w353) -> ("error out"=w357:errorcluster, "refnum out"=w355:T10)  [unwired: 7 in]
            n233 = call <vilib>:"Close Config Data.vi"("error in (no error)"=w357, "refnum"=w355) -> ("error out"=w362:errorcluster, "file path"=w363:path)  [unwired: 8 in]
            n234 = Open/Create/Replace File(file path (use dialog)=w363, error in=w362) -> (refnum out=w359:refnum<file>, error out=w358:errorcluster)  [unwired: 4 in, 1 out]
            n235 = Flush File(refnum=w359, error in=w358) -> (refnum out=w360:refnum<file>, error out=w361:errorcluster)
            n236 = Close File(refnum=w360, error in=w361) -> ()  [unwired: 2 out]
          }
        }
      }
      event "数据发送通道", "数据发送协议", "数据组合发送", "2011发送", "日志、参数发送", "判断数据反馈": Value Change {
        n237 = event-data() -> ("CtlRef"=w367:refnum<vi>, "OldVal"=w365:variant, "NewVal"=w364:variant)  [unwired: 1 in, 3 out]
        n238 = property class="Ctl"(reference=w367) -> ("Label.Text"=w366:string)  [unwired: 1 in, 2 out]
        n239 = case shown="\"数据发送通道\"" w366 {
          tunnel: w365 -> [_ w371 w394 w417 w440 w463 w486]
          tunnel: w364 -> [_ w368 w391 w414 w437 w460 w483]
          frame "假", Default {
          }
          frame "数据发送通道" {
            n240 = Variant To Data(type=enum16{"TCP", "VISA"}."TCP" ("数据发送通道"), Variant=w368) -> (data=w369:enum16{"TCP", "VISA"})  [unwired: 1 in, 1 out]
            n241 = global write "断电保存全局.vi" "数据发送通道"(w369) -> ()
            n242 = Two Button Dialog(message="TCP通过网络发送数据，VISA通过串口发送数据，确定更改数据发送通道吗？" ("消息")) -> (T button?=w372:bool)  [unwired: 2 in]
            n243 = case shown="假" w372 {
              tunnel: w371 -> [w375 _]
              frame False {
                n244 = Variant To Data(type=enum16{"TCP", "VISA"}."TCP" ("数据发送通道"), Variant=w375) -> (data=w374:enum16{"TCP", "VISA"})  [unwired: 1 in, 1 out]
                n245 = global write "断电保存全局.vi" "数据发送通道"(w374) -> ()
              }
              frame True {
                n246 = flat-sequence {
                  frame #0 {
                  }
                  frame #1 {
                    n247 = call <vilib>:"Application Directory.vi"() -> ("Application Directory"=w377:path)
                    n248 = Build Path(base path=w377, name or relative path="data\\sys.ini" ("名称或相对路径")) -> (appended path=w379:path)
                    n249 = call <vilib>:"Open Config Data.vi"("configuration file path"=w379) -> ("error out"=w383:errorcluster, "refnum"=w380:T10)  [unwired: 8 in, 1 out]
                    n250 = vi-ref "断电保存全局.vi"() -> (w381:refnum<vi>)
                    n251 = call <userlib>:"Write Panel to INI__ogtk.vi"("error in (no error)"=w383, "VI ref"=w381, "refnum"=w380) -> ("error out"=w384:errorcluster, "refnum out"=w382:T10)  [unwired: 7 in]
                    n252 = call <vilib>:"Close Config Data.vi"("error in (no error)"=w384, "refnum"=w382) -> ("error out"=w389:errorcluster, "file path"=w390:path)  [unwired: 8 in]
                    n253 = Open/Create/Replace File(file path (use dialog)=w390, error in=w389) -> (refnum out=w386:refnum<file>, error out=w385:errorcluster)  [unwired: 4 in, 1 out]
                    n254 = Flush File(refnum=w386, error in=w385) -> (refnum out=w387:refnum<file>, error out=w388:errorcluster)
                    n255 = Close File(refnum=w387, error in=w388) -> ()  [unwired: 2 out]
                  }
                }
              }
            }
          }
          frame "数据发送协议" {
            n256 = Variant To Data(type=enum16{"2005-212协议", "2017-212协议"}."2017-212协议" ("数据"), Variant=w391) -> (data=w392:enum16{"2005-212协议", "2017-212协议"})  [unwired: 1 in, 1 out]
            n257 = global write "断电保存全局.vi" "数据发送协议"(w392) -> ()
            n258 = Two Button Dialog(message="2005对应旧版通信协议，2017对应最新版协议，对应协议因子编码会不同，\n更改可能导致数据不能被平台识别，确定更改数据发送协议吗？" ("消息")) -> (T button?=w395:bool)  [unwired: 2 in]
            n259 = case shown="真" w395 {
              tunnel: w394 -> [w399 _]
              frame False {
                n260 = Variant To Data(type=enum16{"2005-212协议", "2017-212协议"}."2017-212协议" ("数据"), Variant=w399) -> (data=w397:enum16{"2005-212协议", "2017-212协议"})  [unwired: 1 in, 1 out]
                n261 = global write "断电保存全局.vi" "数据发送协议"(w397) -> ()
              }
              frame True {
                n262 = flat-sequence {
                  frame #0 {
                  }
                  frame #1 {
                    n263 = call <vilib>:"Application Directory.vi"() -> ("Application Directory"=w400:path)
                    n264 = Build Path(base path=w400, name or relative path="data\\sys.ini" ("名称或相对路径")) -> (appended path=w402:path)
                    n265 = call <vilib>:"Open Config Data.vi"("configuration file path"=w402) -> ("error out"=w406:errorcluster, "refnum"=w403:T10)  [unwired: 8 in, 1 out]
                    n266 = vi-ref "断电保存全局.vi"() -> (w404:refnum<vi>)
                    n267 = call <userlib>:"Write Panel to INI__ogtk.vi"("error in (no error)"=w406, "VI ref"=w404, "refnum"=w403) -> ("error out"=w407:errorcluster, "refnum out"=w405:T10)  [unwired: 7 in]
                    n268 = call <vilib>:"Close Config Data.vi"("error in (no error)"=w407, "refnum"=w405) -> ("error out"=w412:errorcluster, "file path"=w413:path)  [unwired: 8 in]
                    n269 = Open/Create/Replace File(file path (use dialog)=w413, error in=w412) -> (refnum out=w409:refnum<file>, error out=w408:errorcluster)  [unwired: 4 in, 1 out]
                    n270 = Flush File(refnum=w409, error in=w408) -> (refnum out=w410:refnum<file>, error out=w411:errorcluster)
                    n271 = Close File(refnum=w410, error in=w411) -> ()  [unwired: 2 out]
                  }
                }
              }
            }
          }
          frame "数据组合发送" {
            n272 = Variant To Data(type=FALSE, Variant=w414) -> (data=w415:bool)  [unwired: 1 in, 1 out]
            n273 = global write "断电保存全局.vi" "数据组合发送"(w415) -> ()
            n274 = Two Button Dialog(message="勾选数据组合发送功能表示所有参数打包整点同时上传、则只能整点发送延时较高，\n不勾选则表示单参数分别上传、则实时性较好，确定更改数据组合发送功能吗？" ("消息")) -> (T button?=w418:bool)  [unwired: 2 in]
            n275 = case shown="假" w418 {
              tunnel: w417 -> [w421 _]
              frame False {
                n276 = Variant To Data(type=FALSE, Variant=w421) -> (data=w420:bool)  [unwired: 1 in, 1 out]
                n277 = global write "断电保存全局.vi" "数据组合发送"(w420) -> ()
              }
              frame True {
                n278 = flat-sequence {
                  frame #0 {
                  }
                  frame #1 {
                    n279 = call <vilib>:"Application Directory.vi"() -> ("Application Directory"=w423:path)
                    n280 = Build Path(base path=w423, name or relative path="data\\sys.ini" ("名称或相对路径")) -> (appended path=w425:path)
                    n281 = call <vilib>:"Open Config Data.vi"("configuration file path"=w425) -> ("error out"=w429:errorcluster, "refnum"=w426:T10)  [unwired: 8 in, 1 out]
                    n282 = vi-ref "断电保存全局.vi"() -> (w427:refnum<vi>)
                    n283 = call <userlib>:"Write Panel to INI__ogtk.vi"("error in (no error)"=w429, "VI ref"=w427, "refnum"=w426) -> ("error out"=w430:errorcluster, "refnum out"=w428:T10)  [unwired: 7 in]
                    n284 = call <vilib>:"Close Config Data.vi"("error in (no error)"=w430, "refnum"=w428) -> ("error out"=w435:errorcluster, "file path"=w436:path)  [unwired: 8 in]
                    n285 = Open/Create/Replace File(file path (use dialog)=w436, error in=w435) -> (refnum out=w432:refnum<file>, error out=w431:errorcluster)  [unwired: 4 in, 1 out]
                    n286 = Flush File(refnum=w432, error in=w431) -> (refnum out=w433:refnum<file>, error out=w434:errorcluster)
                    n287 = Close File(refnum=w433, error in=w434) -> ()  [unwired: 2 out]
                  }
                }
              }
            }
          }
          frame "2011发送" {
            n288 = Variant To Data(type=FALSE, Variant=w437) -> (data=w438:bool)  [unwired: 1 in, 1 out]
            n289 = global write "断电保存全局.vi" "2011发送"(w438) -> ()
            n290 = Two Button Dialog(message="2011表示实时数据上传，一般情况需要勾选，确定更改2011实时数据发送功能吗？" ("消息")) -> (T button?=w441:bool)  [unwired: 2 in]
            n291 = case shown="真" w441 {
              tunnel: w440 -> [w444 _]
              frame False {
                n292 = Variant To Data(type=FALSE, Variant=w444) -> (data=w443:bool)  [unwired: 1 in, 1 out]
                n293 = global write "断电保存全局.vi" "2011发送"(w443) -> ()
              }
              frame True {
                n294 = flat-sequence {
                  frame #0 {
                  }
                  frame #1 {
                    n295 = call <vilib>:"Application Directory.vi"() -> ("Application Directory"=w446:path)
                    n296 = Build Path(base path=w446, name or relative path="data\\sys.ini" ("名称或相对路径")) -> (appended path=w448:path)
                    n297 = call <vilib>:"Open Config Data.vi"("configuration file path"=w448) -> ("error out"=w452:errorcluster, "refnum"=w449:T10)  [unwired: 8 in, 1 out]
                    n298 = vi-ref "断电保存全局.vi"() -> (w450:refnum<vi>)
                    n299 = call <userlib>:"Write Panel to INI__ogtk.vi"("error in (no error)"=w452, "VI ref"=w450, "refnum"=w449) -> ("error out"=w453:errorcluster, "refnum out"=w451:T10)  [unwired: 7 in]
                    n300 = call <vilib>:"Close Config Data.vi"("error in (no error)"=w453, "refnum"=w451) -> ("error out"=w458:errorcluster, "file path"=w459:path)  [unwired: 8 in]
                    n301 = Open/Create/Replace File(file path (use dialog)=w459, error in=w458) -> (refnum out=w455:refnum<file>, error out=w454:errorcluster)  [unwired: 4 in, 1 out]
                    n302 = Flush File(refnum=w455, error in=w454) -> (refnum out=w456:refnum<file>, error out=w457:errorcluster)
                    n303 = Close File(refnum=w456, error in=w457) -> ()  [unwired: 2 out]
                  }
                }
              }
            }
          }
          frame "日志、参数发送" {
            n304 = Variant To Data(type=FALSE, Variant=w460) -> (data=w461:bool)  [unwired: 1 in, 1 out]
            n305 = global write "断电保存全局.vi" "日志、参数发送"(w461) -> ()
            n306 = Two Button Dialog(message="选择是否需要仪器日志、状态和告警信息上传，一般情况需要勾选，确定更改日志、参数发送功能吗？" ("消息")) -> (T button?=w464:bool)  [unwired: 2 in]
            n307 = case shown="真" w464 {
              tunnel: w463 -> [w467 _]
              frame False {
                n308 = Variant To Data(type=FALSE, Variant=w467) -> (data=w466:bool)  [unwired: 1 in, 1 out]
                n309 = global write "断电保存全局.vi" "日志、参数发送"(w466) -> ()
              }
              frame True {
                n310 = flat-sequence {
                  frame #0 {
                  }
                  frame #1 {
                    n311 = call <vilib>:"Application Directory.vi"() -> ("Application Directory"=w469:path)
                    n312 = Build Path(base path=w469, name or relative path="data\\sys.ini" ("名称或相对路径")) -> (appended path=w471:path)
                    n313 = call <vilib>:"Open Config Data.vi"("configuration file path"=w471) -> ("error out"=w475:errorcluster, "refnum"=w472:T10)  [unwired: 8 in, 1 out]
                    n314 = vi-ref "断电保存全局.vi"() -> (w473:refnum<vi>)
                    n315 = call <userlib>:"Write Panel to INI__ogtk.vi"("error in (no error)"=w475, "VI ref"=w473, "refnum"=w472) -> ("error out"=w476:errorcluster, "refnum out"=w474:T10)  [unwired: 7 in]
                    n316 = call <vilib>:"Close Config Data.vi"("error in (no error)"=w476, "refnum"=w474) -> ("error out"=w481:errorcluster, "file path"=w482:path)  [unwired: 8 in]
                    n317 = Open/Create/Replace File(file path (use dialog)=w482, error in=w481) -> (refnum out=w478:refnum<file>, error out=w477:errorcluster)  [unwired: 4 in, 1 out]
                    n318 = Flush File(refnum=w478, error in=w477) -> (refnum out=w479:refnum<file>, error out=w480:errorcluster)
                    n319 = Close File(refnum=w479, error in=w480) -> ()  [unwired: 2 out]
                  }
                }
              }
            }
          }
          frame "判断数据反馈" {
            n320 = Variant To Data(type=FALSE, Variant=w483) -> (data=w484:bool)  [unwired: 1 in, 1 out]
            n321 = global write "断电保存全局.vi" "判断数据反馈"(w484) -> ()
            n322 = Two Button Dialog(message="勾选判断数据反馈是针对平台能有反馈的情况、此功能能保证数据的完整性，尽可能的防止各种问题导致的数据缺失，\n不勾选则表示数据只发送不判断平台的反馈、用于针对平台没有反馈的情况，确定更改判断数据反馈功能吗？" ("消息")) -> (T button?=w487:bool)  [unwired: 2 in]
            n323 = case shown="真" w487 {
              tunnel: w486 -> [w490 _]
              frame False {
                n324 = Variant To Data(type=FALSE, Variant=w490) -> (data=w489:bool)  [unwired: 1 in, 1 out]
                n325 = global write "断电保存全局.vi" "判断数据反馈"(w489) -> ()
              }
              frame True {
                n326 = flat-sequence {
                  frame #0 {
                  }
                  frame #1 {
                    n327 = call <vilib>:"Application Directory.vi"() -> ("Application Directory"=w492:path)
                    n328 = Build Path(base path=w492, name or relative path="data\\sys.ini" ("名称或相对路径")) -> (appended path=w494:path)
                    n329 = call <vilib>:"Open Config Data.vi"("configuration file path"=w494) -> ("error out"=w498:errorcluster, "refnum"=w495:T10)  [unwired: 8 in, 1 out]
                    n330 = vi-ref "断电保存全局.vi"() -> (w496:refnum<vi>)
                    n331 = call <userlib>:"Write Panel to INI__ogtk.vi"("error in (no error)"=w498, "VI ref"=w496, "refnum"=w495) -> ("error out"=w499:errorcluster, "refnum out"=w497:T10)  [unwired: 7 in]
                    n332 = call <vilib>:"Close Config Data.vi"("error in (no error)"=w499, "refnum"=w497) -> ("error out"=w504:errorcluster, "file path"=w505:path)  [unwired: 8 in]
                    n333 = Open/Create/Replace File(file path (use dialog)=w505, error in=w504) -> (refnum out=w501:refnum<file>, error out=w500:errorcluster)  [unwired: 4 in, 1 out]
                    n334 = Flush File(refnum=w501, error in=w500) -> (refnum out=w502:refnum<file>, error out=w503:errorcluster)
                    n335 = Close File(refnum=w502, error in=w503) -> ()  [unwired: 2 out]
                  }
                }
              }
            }
          }
        }
      }
      event "确定": Value Change {
        n336 = event-data() -> ()  [unwired: 1 in, 6 out]
        n337 = call "通信状态入队列.vi"("枚举"=enum16{"打开连接", "发送数据", "读取数据", "数据处理", "关闭连接"}."关闭连接") -> ()  [unwired: 10 in, 1 out]
      }
      event "参数配置": Value Change {
        n338 = event-data() -> ()  [unwired: 1 in, 6 out]
        n339 = property on="窗格" class="Pane"("Origin"=T8 {"Horizontal"=0, "Vertical"=1000} ("原点")) -> ()  [unwired: 2 in, 2 out]
      }
      event "返回": Value Change {
        n340 = event-data() -> ()  [unwired: 1 in, 6 out]
        n341 = property on="窗格" class="Pane"("Origin"=T8 {"Horizontal"=0, "Vertical"=0} ("原点")) -> ()  [unwired: 2 in, 2 out]
      }
      event "确定更改起始时间": Value Change {
        n342 = event-data() -> ()  [unwired: 1 in, 6 out]
        n343 = local write "更改起始时间"(FALSE ("更改起始时间")) -> ()
        n344 = Two Button Dialog(message="确定以当前设置时间作为数据索引起始时间？" ("消息")) -> (T button?=w509:bool)  [unwired: 2 in]
        n345 = case shown="真" w509 {
          frame False {
          }
          frame True {
            n346 = global write "断电保存全局.vi" "数据重发"(TRUE ("数据重发")) -> ()
            n347 = Format Date/Time String(time format string (%c)="%Y/%m/%d %H:%M:%S" ("时间格式字符串(%c)"), seconds (now)="数据发送起始时间") -> (date/time string=w513:string)  [unwired: 1 in]
            n348 = global write "断电保存全局.vi" "数据重发时间戳"(w513) -> ()
            n349 = Initialize Array(w513, 27 ("维数大小")) -> (w514:string[])
            n350 = Array To Cluster(array=w514) -> (cluster=w512:T12)
            n351 = global write "全局 水样时间.vi" "水样数据索引"(w512) -> ()
            n352 = global read "断电保存全局.vi" "数据组合发送"() -> (w518:bool)
            n353 = case shown="假" w518 {
              tunnel: w513 -> [w520 _]
              frame False {
                n354 = global write "全局 时间2.vi" "标样核查索引起始时间"(w520) -> ()
                n355 = global write "全局 时间2.vi" "加标回收索引起始时间"(w520) -> ()
                n356 = global write "全局 时间2.vi" "跨度核查索引起始时间"(w520) -> ()
                n357 = global write "全局 时间2.vi" "零点核查索引起始时间"(w520) -> ()
                n358 = Initialize Array(w520, 8 ("维数大小")) -> (w526:string[])
                n359 = Initialize Array(w520, 15 ("维数大小")) -> (w521:string[])
                n360 = Array To Cluster(array=w526) -> (cluster=w525:T14)
                n361 = Array To Cluster(array=w521) -> (cluster=w522:T15)
                n362 = global write "全局 时间2.vi" "零点核查索引"(w525) -> ()
                n363 = global write "全局 时间2.vi" "跨度核查索引"(w525) -> ()
                n364 = global write "全局 时间2.vi" "标样核查索引"(w522) -> ()
                n365 = global write "全局 时间2.vi" "集成干预索引"(w522) -> ()
              }
              frame True {
              }
            }
          }
        }
      }
      event "开机启动": Value Change {
        n366 = event-data() -> ("NewVal"=w527:bool)  [unwired: 1 in, 5 out]
        n367 = case shown="假" w527 {
          frame False {
            n368 = Two Button Dialog(message="是否删除开机启动？" ("消息"), 1:"否" ("F按钮名称（“取消”）"), 2:"是" ("T按钮名称（“确定”）")) -> (T button?=w528:bool)
            n369 = case shown="真" w528 {
              frame False {
              }
              frame True {
                n370 = call <vilib>:"Application Directory.vi"() -> ("Application Directory"=w533:path)
                n371 = call "删除启动项.vi"("启动文件路径"=w533) -> ("删除标记"=w532:bool)  [unwired: 9 in, 1 out]
                n372 = case shown="假" w532 {
                  tunnel: ["删除开机启动失败" ("T按钮名称（“确定”）") "删除开机启动成功" ("T按钮名称（“确定”）")] -> w534
                  frame False {
                  }
                  frame True {
                  }
                }
                n373 = One Button Dialog(message=w534) -> ()  [unwired: 1 in, 1 out]
              }
            }
          }
          frame True {
            n374 = Two Button Dialog(message="是否添加开机启动？" ("消息"), 1:"否" ("F按钮名称（“取消”）"), 2:"是" ("T按钮名称（“确定”）")) -> (T button?=w537:bool)
            n375 = case shown="真" w537 {
              frame False {
              }
              frame True {
                n376 = call <vilib>:"Application Directory.vi"() -> ("Application Directory"=w543:path)
                n377 = call "添加启动项.vi"("启动文件路径"=w543) -> ("添加成功标记"=w542:bool)  [unwired: 9 in, 1 out]
                n378 = case shown="真" w542 {
                  tunnel: ["添加开机启动失败" ("T按钮名称（“确定”）") "添加开机启动成功" ("T按钮名称（“确定”）")] -> w541
                  frame False {
                  }
                  frame True {
                  }
                }
                n379 = One Button Dialog(message=w541) -> ()  [unwired: 1 in, 1 out]
              }
            }
          }
        }
      }
      event "更新": Value Change {
        n380 = event-data() -> ()  [unwired: 1 in, 6 out]
        n381 = call "自定义双按钮对话框.vi"("消息"="选择是否从服务器获取最新版本信息？") -> ("输出"=w546:bool)  [unwired: 10 in]
        n382 = case shown="真" w546 {
          frame False {
          }
          frame True {
            # "获取最新版本"
            n383 = disable-structure shown="禁用" {
              frame Disabled {
                n384 = call "FTP自动升级更新main.vi"() -> ()  [unwired: 12 in]
              }
              frame Enabled {
              }
            }
          }
        }
      }
      event "updateconfiguration": Value Change {
        n385 = event-data() -> ("NewVal"=w555:T1)  [unwired: 1 in, 5 out]
        n386 = call <vilib>:"Application Directory.vi"() -> ("Application Directory"=w559:path)
        n387 = Build Array("主机" ("section"), "用户" ("section"), "密码" ("key"), "远程路径" ("key"), "下载文件名" ("key"), "软件版本" ("key")) -> (w548:string[])
        n388 = Build Path(base path=w559, name or relative path="update\\data\\set.ini" ("名称或相对路径")) -> (appended path=w557:path)
        n389 = call "配置文件write.vi"("updateconfiguration"=w555, "configuration file path"=w557, "键数组"=w548, "段"="应用程序交互" ("section")) -> ("error out"=w556:errorcluster)  [unwired: 7 in]
        n390 = call <vilib>:"Clear Errors.vi"("error in (no error)"=w556) -> ()  [unwired: 5 in, 2 out]
      }
      event "IP", "PORT": Mouse Down {
        n391 = event-data() -> ("CtlRef"=w564:refnum<vi>)  [unwired: 1 in, 7 out]
        n392 = property class="Str"(reference=w564) -> (reference out=w562:refnum<vi>, "Value"=w563:string)  [unwired: 1 in, 1 out]
        n393 = call "IP键盘.vi"("OldNumber"=w563) -> ("NewNumber"=w561:string)
        n394 = property class="Str"(reference=w562, "Val(Sgnl)"=w561) -> ()  [unwired: 1 in, 2 out]
      }
    }
  }
  n395 = disable-structure shown="启用" {
    disable-tunnel: [w566 T16."Standard" ("状态")] -> w69
    disable-tunnel: w46 -> [w565 _]
    frame Disabled {
      n396 = case shown="\"Development System\", 默认" w565 {
        tunnel: [T16."Standard" ("状态") T16."Hidden" ("状态")] -> w566
        frame "Development System", Default {
        }
        frame "Run Time System" {
        }
      }
    }
    frame Enabled {
    }
  }
  n397 = Obtain Queue(name (unnamed)="actualwrite" ("名称（未命名）"), element data type=enum16{"打开连接", "发送数据", "读取数据", "数据处理", "关闭连接"}."打开连接" ("枚举")) -> (queue out=w25:refnum<queue>, error out=w24:errorcluster)  [unwired: 3 in, 1 out]
  n398 = Obtain Queue(name (unnamed)="actualread" ("名称（未命名）"), element data type=enum16{"打开连接", "发送数据", "读取数据", "数据处理", "关闭连接"}."打开连接" ("枚举")) -> (queue out=w22:refnum<queue>, error out=w15:errorcluster)  [unwired: 3 in, 1 out]
  n399 = property class="VI"(reference=w37) -> ("Name"=w36:string)  [unwired: 1 in, 2 out]
  n400 = property class="VI"(reference=w38) -> ("Name"=w45:string)  [unwired: 1 in, 2 out]
  n401 = while {
    tunnel: w25 -> [w578]
    tunnel: w24 -> [w577]
    shift-right: [w573] -> _
    shift-left: errorcluster {"status"=FALSE, "code"=0, "source"=""} ("error out") -> [w572]
    stop <- FALSE stop-if-true
    # "写入数据出队列"
    n402 = Dequeue Element(queue=w578, timeout in ms (-1)=30000 ("超时毫秒(-1)"), error in (no error)=w577) -> (queue out=w571:refnum<queue>, element=w575:enum16{"打开连接", "发送数据", "读取数据", "数据处理", "关闭连接"}, timed out?=w574:bool, error out=w570:errorcluster)
    n403 = case shown="无错误" w572 {
      tunnel: w575 -> [w580 _]
      tunnel: w574 -> [w582 _]
      tunnel: [w586 w627] -> w573
      tunnel: w572 -> [w585 w631]
      tunnel: w571 -> [w584 w629]
      tunnel: w570 -> [w583 w628]
      frame No Error {
        n404 = case shown="真" w582 {
          tunnel: [w587 enum16{"打开连接", "发送数据", "读取数据", "数据处理", "关闭连接"}."发送数据" ("枚举")] -> w581
          tunnel: w580 -> [w587 _]
          frame False {
          }
          frame True {
          }
        }
        n405 = case shown="\"发送数据\", 默认" w581 {
          tunnel: w582 -> [_ w604 _ _ _]
          tunnel: [w590 w599 _ _ w620] -> w586
          tunnel: w585 -> [w592 w606 _ _ w621]
          tunnel: w584 -> [_ _ _ _ w622]
          tunnel: w583 -> [_ _ _ _ w619]
          frame "打开连接" {
            n406 = global read "断电保存全局.vi" "VISA resource name"() -> (w598:refnum<visa-resource-name>)
            n407 = global read "断电保存全局.vi" "数据发送通道"() -> (w595:enum16{"TCP", "VISA"})
            n408 = global read "断电保存全局.vi" "baud rate"() -> (w597:u32)
            n409 = global read "断电保存全局.vi" "PORT"() -> (w596:string)
            n410 = global read "断电保存全局.vi" "IP"() -> (w594:string)
            n411 = call "VISATCP组合选择发送.vi"("IP"=w594, "数据发送通道"=w595, "命令"="open", "PORT"=w596, "VISA resource name"=w598, "baud rate"=w597, "error in (no error)"=w592) -> ("错误输出"=w590:errorcluster)  [unwired: 5 in, 3 out]
            n412 = Unbundle By Name(w590) -> ("status"=w589:bool)  [unwired: 1 out]
            n413 = Not(x=w589) -> (.not. x?=w591:bool)
            n414 = global write "全局 数据发送重叠.vi" "掉线指示灯"(w589) -> ()
            n415 = local write "通信状态"(w591) -> ()
          }
          frame "发送数据", Default {
            n416 = case shown="真" w604 {
              tunnel: [w611 w613] -> w601
              tunnel: w606 -> [w610 w614]
              tunnel: [w610 w614] -> w605
              frame False {
                # "事件触发发送数据"
                n417 = global read "全局1.vi" "发送报文显示"() -> (w611:string)
              }
              frame True {
                # "30秒超时发送心跳包"
                n418 = local read "配置信息"() -> (w617:T5)
                n419 = Unbundle By Name(w617) -> ("MN"=w616:string, "PW"=w615:string)
                n420 = call "数据编码.vi"("table输入"="心跳包", "MN"=w616, "PW"=w615) -> ("通讯包字符串"=w613:string)  [unwired: 11 in, 1 out]
                n421 = global write "全局1.vi" "发送报文显示"(w613) -> ()
                n422 = Wait (ms)(milliseconds to wait=u32 500 ("等待时间（毫秒）")) -> ()  [unwired: 1 out]
              }
            }
            n423 = global read "断电保存全局.vi" "数据发送通道"() -> (w607:enum16{"TCP", "VISA"})
            n424 = Concatenate Strings("send:" ("字符串"), w601) -> (w600:string)
            n425 = call "VISATCP组合选择发送.vi"("数据发送通道"=w607, "命令"="write", "error in (no error)"=w605, "写入缓冲区"=w601) -> ("错误输出"=w599:errorcluster)  [unwired: 8 in, 3 out]
            n426 = Build Array(w600) -> (w603:string[])
            n427 = call "发送数据记录到文档(子VI).vi"("数组"=w603) -> ()  [unwired: 9 in, 1 out]
            n428 = flat-sequence {
              tunnel: w599 -> [_]
              frame #0 {
                n429 = local write "心跳包"(FALSE ("心跳包")) -> ()
              }
            }
            "心跳包" <- w604
          }
          frame "读取数据" {
          }
          frame "数据处理" {
          }
          frame "关闭连接" {
            n430 = global read "断电保存全局.vi" "数据发送通道"() -> (w624:enum16{"TCP", "VISA"})
            n431 = Enqueue Element(queue=w622, element=enum16{"打开连接", "发送数据", "读取数据", "数据处理", "关闭连接"}."打开连接" ("枚举"), error in (no error)=w619) -> ()  [unwired: 1 in, 3 out]
            n432 = call "VISATCP组合选择发送.vi"("数据发送通道"=w624, "命令"="close", "error in (no error)"=w621) -> ("错误输出"=w625:errorcluster)  [unwired: 9 in, 3 out]
            n433 = call <vilib>:"Clear Errors.vi"("error in (no error)"=w625) -> ("error out"=w620:errorcluster)  [unwired: 5 in, 1 out]
          }
        }
      }
      frame Error {
        n434 = Unbundle By Name(w631) -> ("code"=w630:i32)
        n435 = case shown="0, 默认" w630 {
          tunnel: w629 -> [w638 w654 w666]
          tunnel: w628 -> [w637 w653 w665]
          tunnel: [w636 w651 w664] -> w627
          frame 0, Default {
            n436 = Flush Queue(queue=w638, error in (no error)=w637) -> (queue out=w640:refnum<queue>, error out=w641:errorcluster)  [unwired: 1 out]
            n437 = local read "状态信息"() -> (w635:T4)
            n438 = Unbundle By Name(w635) -> ("TCP服务端掉线计数"=w633:i32)
            n439 = Enqueue Element(queue=w640, element=enum16{"打开连接", "发送数据", "读取数据", "数据处理", "关闭连接"}."关闭连接" ("枚举"), error in (no error)=w641) -> (error out=w642:errorcluster)  [unwired: 1 in, 2 out]
            n440 = Increment(x=w633) -> (x+1=w634:i32)
            n441 = Bundle By Name(cluster=w635, "TCP服务端掉线计数"=w634) -> (w632:T4)
            n442 = local write "状态信息"(w632) -> ()
            n443 = call <vilib>:"Clear Errors.vi"("error in (no error)"=w642) -> ("error out"=w636:errorcluster)  [unwired: 5 in, 1 out]
          }
          frame 54, 63 {
            n444 = Flush Queue(queue=w654, error in (no error)=w653) -> (queue out=w656:refnum<queue>, error out=w657:errorcluster)  [unwired: 1 out]
            n445 = local read "状态信息"() -> (w646:T4)
            n446 = Unbundle By Name(w646) -> ("TCP服务端掉线计数"=w650:i32, "TCP掉线时间节点"=w643:string)
            n447 = Enqueue Element(queue=w656, element=enum16{"打开连接", "发送数据", "读取数据", "数据处理", "关闭连接"}."关闭连接" ("枚举"), error in (no error)=w657) -> (error out=w652:errorcluster)  [unwired: 1 in, 2 out]
            n448 = Less Or Equal?(x=w650, y=1) -> (x <= y?=w648:bool)
            n449 = case shown="真" w648 {
              tunnel: [w658 w659] -> w647
              tunnel: w643 -> [w658 _]
              frame False {
              }
              frame True {
                n450 = Get Date/Time In Seconds() -> (seconds since 1Jan1904=w660:timestamp)
                n451 = Format Date/Time String(time format string (%c)="%Y%m%d%H%M%S%3u" ("时间格式字符串(%c)"), seconds (now)=w660) -> (date/time string=w662:string)  [unwired: 1 in]
                n452 = call "格式时间字符串.vi"("字符串"=w662) -> ("连接的字符串"=w659:string)  [unwired: 10 in]
              }
            }
            n453 = Increment(x=w650) -> (x+1=w645:i32)
            n454 = call <vilib>:"Clear Errors.vi"("error in (no error)"=w652) -> ("error out"=w651:errorcluster)  [unwired: 5 in, 1 out]
            n455 = Bundle By Name(cluster=w646, "TCP服务端掉线计数"=w645, "TCP掉线时间节点"=w647) -> (w644:T4)
            n456 = local write "状态信息"(w644) -> ()
          }
          frame 56 {
            n457 = Flush Queue(queue=w666, error in (no error)=w665) -> (error out=w663:errorcluster)  [unwired: 2 out]
            n458 = call <vilib>:"Clear Errors.vi"("error in (no error)"=w663) -> ("error out"=w664:errorcluster)  [unwired: 5 in, 1 out]
          }
        }
      }
    }
  }
  n459 = call <vilib>:"Application Directory.vi"() -> ("Application Directory"=w52:path)
  n460 = property class="App"() -> ("App.Name"=w4:string)  [unwired: 2 in, 2 out]
  n461 = Open VI Reference(type specifier VI Refnum (for type only)=refnum<vi> refnum, vi path=w36, options=128 ("选项")) -> (vi reference=w34:refnum<vi>, error out=w32:errorcluster)  [unwired: 3 in]
  n462 = Open VI Reference(type specifier VI Refnum (for type only)=refnum<vi> refnum, vi path=w45, options=128 ("选项")) -> (vi reference=w43:refnum<vi>, error out=w41:errorcluster)  [unwired: 3 in]
  n463 = Obtain Queue(name (unnamed)="反控命令信息队列" ("名称（未命名）"), element data type=cluster{"命令编码CN":string, "QN":string} {"命令编码CN"="", "QN"=""}) -> (queue out=w9:refnum<queue>, error out=w8:errorcluster)  [unwired: 3 in, 1 out]
  n464 = Build Path(base path=w52, name or relative path="data\\tubiao.ico" ("名称或相对路径")) -> (appended path=w60:path)
  n465 = Enqueue Element(queue=w22, element=enum16{"打开连接", "发送数据", "读取数据", "数据处理", "关闭连接"}."打开连接" ("枚举"), error in (no error)=w15) -> (queue out=w18:refnum<queue>, error out=w17:errorcluster)  [unwired: 1 in, 1 out]
  n466 = Obtain Queue(name (unnamed)="datasent" ("名称（未命名）"), element data type="实时小时数据" ("元素")) -> (queue out=w13:refnum<queue>, error out=w12:errorcluster)  [unwired: 3 in, 1 out]
  n467 = Current VI's Path() -> (path=w49:path)
  n468 = call-by-ref "?"(reference=w34, error in=w32) -> (reference out=w30:refnum<vi>, error out=w31:errorcluster)  [unwired: 12 in]
  n469 = call-by-ref "?"(reference=w43, error in=w41) -> (reference out=w39:refnum<vi>, error out=w40:errorcluster)  [unwired: 12 in]
  n470 = Build Array(w60) -> (w55:path[])
  n471 = Open VI Reference(vi path=w49) -> (vi reference=w48:refnum<vi>)  [unwired: 5 in, 1 out]
  n472 = Close Reference(reference=w30, error in (no error)=w31) -> ()  [unwired: 1 out]
  n473 = Close Reference(reference=w39, error in (no error)=w40) -> ()  [unwired: 1 out]
  n474 = invoke class="VI" method="FP.Open"(reference=w48, "Activate"=TRUE ("激活？"), "State"=w69) -> (error out=w47:errorcluster)  [unwired: 2 in, 4 out]
  n475 = while {
    tunnel: w18 -> [w679]
    tunnel: w17 -> [w678]
    shift-right: [w675] -> _
    shift-left: errorcluster {"status"=FALSE, "code"=0, "source"=""} ("error out") -> [w674]
    tunnel: w13 -> [w670]
    tunnel: w12 -> [w669]
    tunnel: w9 -> [w668]
    tunnel: w8 -> [w667]
    stop <- FALSE stop-if-true
    # "读取数据出队列处理"
    n476 = Dequeue Element(queue=w679, error in (no error)=w678) -> (queue out=w673:refnum<queue>, element=w676:enum16{"打开连接", "发送数据", "读取数据", "数据处理", "关闭连接"}, error out=w672:errorcluster)  [unwired: 1 in, 1 out]
    n477 = Wait (ms)(milliseconds to wait=u32 1000 ("等待时间（毫秒）")) -> ()  [unwired: 1 out]
    n478 = case shown="无错误" w674 {
      tunnel: w676 -> [w685 _]
      tunnel: [w692 w770] -> w675
      tunnel: w674 -> [w691 w774]
      tunnel: w673 -> [w690 w772]
      tunnel: w672 -> [w689 w771]
      tunnel: w670 -> [w683 _]
      tunnel: w669 -> [w682 _]
      tunnel: w668 -> [w681 _]
      tunnel: w667 -> [w680 _]
      frame No Error {
        n479 = case shown="\"打开连接\", 默认" w685 {
          tunnel: [w699 _ w733 _ w765] -> w692
          tunnel: w691 -> [w698 _ w736 _ w766]
          tunnel: w690 -> [w696 _ w728 _ w763]
          tunnel: w689 -> [w695 _ w727 _ w762]
          tunnel: [w694 _ _ _ _] -> w686
          tunnel: w683 -> [_ _ w720 _ _]
          tunnel: w682 -> [_ _ w719 _ _]
          tunnel: w681 -> [_ _ w708 _ _]
          tunnel: w680 -> [_ _ w707 _ _]
          frame "打开连接", Default {
            n480 = Enqueue Element(queue=w696, element=enum16{"打开连接", "发送数据", "读取数据", "数据处理", "关闭连接"}."读取数据" ("枚举"), error in (no error)=w695) -> ()  [unwired: 1 in, 3 out]
            n481 = global read "断电保存全局.vi" "VISA resource name"() -> (w706:refnum<visa-resource-name>)
            n482 = global read "断电保存全局.vi" "数据发送通道"() -> (w703:enum16{"TCP", "VISA"})
            n483 = global read "断电保存全局.vi" "baud rate"() -> (w705:u32)
            n484 = global read "断电保存全局.vi" "PORT"() -> (w704:string)
            n485 = global read "断电保存全局.vi" "IP"() -> (w702:string)
            n486 = call "VISATCP组合选择发送.vi"("IP"=w702, "数据发送通道"=w703, "命令"="open", "PORT"=w704, "VISA resource name"=w706, "baud rate"=w705, "error in (no error)"=w698) -> ("错误输出"=w699:errorcluster)  [unwired: 5 in, 3 out]
            n487 = Unbundle By Name(w699) -> ("status"=w693:bool, "code"=w694:i32)
            n488 = Not(x=w693) -> (.not. x?=→"通信状态":bool)
            n489 = global write "全局 数据发送重叠.vi" "掉线指示灯"(w693) -> ()
          }
          frame "发送数据" {
          }
          frame "读取数据" {
            n490 = Get Queue Status(queue=w728, error in (no error)=w727) -> (queue out=w724:refnum<queue>, error out=w723:errorcluster, # elements in queue=w726:i32)  [unwired: 1 in, 5 out]
            n491 = global read "断电保存全局.vi" "数据发送通道"() -> (w735:enum16{"TCP", "VISA"})
            n492 = Equal To 0?(x=w726) -> (x = 0?=w725:bool)
            n493 = case shown="真" w725 {
              tunnel: w724 -> [_ w760]
              tunnel: w723 -> [_ w759]
              frame False {
              }
              frame True {
                n494 = Enqueue Element(queue=w760, element=enum16{"打开连接", "发送数据", "读取数据", "数据处理", "关闭连接"}."读取数据" ("枚举"), error in (no error)=w759) -> ()  [unwired: 1 in, 3 out]
              }
            }
            n495 = call "VISATCP组合选择发送.vi"("数据发送通道"=w735, "命令"="read", "error in (no error)"=w736) -> ("读取缓冲区"=w721:string, "错误输出"=w733:errorcluster)  [unwired: 9 in, 2 out]
            n496 = call "读取数据处理 (子VI).vi"("data out"=w721) -> ("命令编码CN"=w729:string, "数据"=w717:string, "时间QN"=w709:string)  [unwired: 8 in, 4 out]
            n497 = Empty String/Path?(string/path=w721) -> (empty?=w722:bool)
            n498 = case shown="假" w722 {
              tunnel: w721 -> [w756 _]
              tunnel: w709 -> [w753 _]
              frame False {
                n499 = Search/Split String(string=w753, search string/char (-)="QN=" ("搜索字符串/字符(-)")) -> (match + rest of string=w752:string)  [unwired: 1 in, 2 out]
                n500 = global write "全局1.vi" "数据输出"(w756) -> ()
                n501 = global write "全局1.vi" "读取报文显示"(w756) -> ()
                n502 = String Subset(string=w752, offset (0)=3 ("偏移量(0)")) -> (substring=w751:string)  [unwired: 1 in]
                n503 = global write "全局1.vi" "QN"(w751) -> ()
                n504 = call "数据记录.vi"("写入字段"=w756) -> ("连接的字符串"=w757:string)  [unwired: 10 in]
                n505 = Build Array(w757) -> (w758:string[])
                n506 = call "发送数据记录到文档(子VI).vi"("数组"=w758) -> ()  [unwired: 9 in, 1 out]
              }
              frame True {
              }
            }
            n507 = Search/Split String(string=w729, search string/char (-)="CN=" ("搜索字符串/字符(-)")) -> (match + rest of string=w730:string)  [unwired: 1 in, 2 out]
            n508 = String Subset(string=w730, offset (0)=3 ("偏移量(0)")) -> (substring=w715:string)  [unwired: 1 in]
            n509 = Empty String/Path?(string/path=w715) -> (empty?=w718:bool)
            n510 = Not Equal?(x=w715, y="9013") -> (x != y?=w712:bool)
            n511 = Not Equal?(x=w715, y="9014") -> (x != y?=w711:bool)
            n512 = Not(x=w718) -> (.not. x?=w710:bool)
            n513 = Compound Arithmetic op=AND ("复合运算")(w710, w712, w711) -> (w716:bool)
            n514 = case shown="真" w716 {
              tunnel: w720 -> [_ w750]
              tunnel: w719 -> [_ w749]
              tunnel: w717 -> [_ w748]
              tunnel: w715 -> [_ w739]
              tunnel: w709 -> [_ w744]
              tunnel: w708 -> [_ w743]
              tunnel: w707 -> [_ w742]
              frame False {
              }
              frame True {
                n515 = global write "全局1.vi" "数据"(w748) -> ()
                n516 = Search/Split String(string=w744, search string/char (-)="QN=" ("搜索字符串/字符(-)")) -> (match + rest of string=w747:string)  [unwired: 1 in, 2 out]
                n517 = global write "全局1.vi" "命令编码CN"(w739) -> ()
                n518 = String Subset(string=w747, offset (0)=3 ("偏移量(0)")) -> (substring=w738:string)  [unwired: 1 in]
                n519 = Bundle By Name(cluster=cluster{"命令编码CN":string, "QN":string} {"命令编码CN"="", "QN"=""}, "命令编码CN"=w739, "QN"=w738) -> (w740:cluster{"命令编码CN":string, "QN":string})
                n520 = Enqueue Element At Opposite End(queue=w750, element="反控命令" ("元素"), error in (no error)=w749) -> ()  [unwired: 1 in, 3 out]
                n521 = Enqueue Element(queue=w743, element=w740, error in (no error)=w742) -> ()  [unwired: 1 in, 3 out]
              }
            }
          }
          frame "数据处理" {
          }
          frame "关闭连接" {
            n522 = global read "断电保存全局.vi" "数据发送通道"() -> (w768:enum16{"TCP", "VISA"})
            n523 = Enqueue Element(queue=w763, element=enum16{"打开连接", "发送数据", "读取数据", "数据处理", "关闭连接"}."打开连接" ("枚举"), error in (no error)=w762) -> ()  [unwired: 1 in, 3 out]
            n524 = call "VISATCP组合选择发送.vi"("数据发送通道"=w768, "命令"="close", "error in (no error)"=w766) -> ("错误输出"=w767:errorcluster)  [unwired: 9 in, 3 out]
            n525 = call <vilib>:"Clear Errors.vi"("error in (no error)"=w767) -> ("error out"=w765:errorcluster)  [unwired: 5 in, 1 out]
          }
        }
        n526 = local read "状态信息"() -> (w688:T4)
        n527 = Bundle By Name(cluster=w688, "TCP服务端掉线计数"=0, "1st Error to Convert"=w686, "步骤"=w685) -> (→"状态信息":T4)
      }
      frame Error {
        n528 = Unbundle By Name(w774) -> ("code"=w773:i32)
        n529 = case shown="54, 63" w773 {
          tunnel: w772 -> [w781 w797 w808]
          tunnel: w771 -> [w780 w796 w807]
          tunnel: [w779 w794 w806] -> w770
          frame 0, Default {
            n530 = Flush Queue(queue=w781, error in (no error)=w780) -> (queue out=w783:refnum<queue>, error out=w784:errorcluster)  [unwired: 1 out]
            n531 = local read "状态信息"() -> (w778:T4)
            n532 = Enqueue Element(queue=w783, element=enum16{"打开连接", "发送数据", "读取数据", "数据处理", "关闭连接"}."关闭连接" ("枚举"), error in (no error)=w784) -> (error out=w785:errorcluster)  [unwired: 1 in, 2 out]
            n533 = Unbundle By Name(w778) -> ("TCP服务端掉线计数"=w776:i32)
            n534 = Increment(x=w776) -> (x+1=w777:i32)
            n535 = Bundle By Name(cluster=w778, "TCP服务端掉线计数"=w777) -> (w775:T4)
            n536 = local write "状态信息"(w775) -> ()
            n537 = call <vilib>:"Clear Errors.vi"("error in (no error)"=w785) -> ("error out"=w779:errorcluster)  [unwired: 5 in, 1 out]
          }
          frame 54, 63 {
            n538 = Flush Queue(queue=w797, error in (no error)=w796) -> (queue out=w799:refnum<queue>, error out=w800:errorcluster)  [unwired: 1 out]
            n539 = local read "状态信息"() -> (w789:T4)
            n540 = Unbundle By Name(w789) -> ("TCP服务端掉线计数"=w793:i32, "TCP掉线时间节点"=w786:string)
            n541 = Enqueue Element(queue=w799, element=enum16{"打开连接", "发送数据", "读取数据", "数据处理", "关闭连接"}."关闭连接" ("枚举"), error in (no error)=w800) -> (error out=w795:errorcluster)  [unwired: 1 in, 2 out]
            n542 = Less Or Equal?(x=w793, y=1) -> (x <= y?=w791:bool)
            n543 = Increment(x=w793) -> (x+1=w788:i32)
            n544 = case shown="真" w791 {
              tunnel: [w801 w802] -> w790
              tunnel: w786 -> [w801 _]
              frame False {
              }
              frame True {
                n545 = Get Date/Time In Seconds() -> (seconds since 1Jan1904=w803:timestamp)
                n546 = Format Date/Time String(time format string (%c)="%Y%m%d%H%M%S%3u" ("时间格式字符串(%c)"), seconds (now)=w803) -> (date/time string=w805:string)  [unwired: 1 in]
                n547 = call "格式时间字符串.vi"("字符串"=w805) -> ("连接的字符串"=w802:string)  [unwired: 10 in]
              }
            }
            n548 = call <vilib>:"Clear Errors.vi"("error in (no error)"=w795) -> ("error out"=w794:errorcluster)  [unwired: 5 in, 1 out]
            n549 = Bundle By Name(cluster=w789, "TCP服务端掉线计数"=w788, "TCP掉线时间节点"=w790) -> (w787:T4)
            n550 = local write "状态信息"(w787) -> ()
          }
          frame 56 {
            n551 = Flush Queue(queue=w808, error in (no error)=w807) -> (queue out=w810:refnum<queue>, error out=w811:errorcluster)  [unwired: 1 out]
            n552 = Enqueue Element(queue=w810, element=enum16{"打开连接", "发送数据", "读取数据", "数据处理", "关闭连接"}."读取数据" ("枚举"), error in (no error)=w811) -> (error out=w812:errorcluster)  [unwired: 1 in, 2 out]
            n553 = call <vilib>:"Clear Errors.vi"("error in (no error)"=w812) -> ("error out"=w806:errorcluster)  [unwired: 5 in, 1 out]
          }
        }
      }
    }
  }
  n554 = Build Array("Open", w4, "Exit" ("元素")) -> (w2:string[])
  n555 = call <vilib>:"Constructor.vi"("error in"=w47, "IconFilePathList"=w55) -> ("error out"=w59:errorcluster, "NotifyIcon"=w53:refnum<class "NotifyIcon.lvclass">)  [unwired: 8 in]
  n556 = for {
    shift-right: [w817] -> w71
    shift-left: w59 -> [w818]
    tunnel: w2 -> [w816] mode=indexing
    tunnel: w1 -> [w815] mode=indexing
    shift-right: [w813] -> w70
    shift-left: w53 -> [w814]
    # "2."
    n557 = call <vilib>:"InsertMenuItem.vi"("error in"=w818, "ItemTag"=w815, "ItemName"=w816, "NotifyIcon in"=w814) -> ("error out"=w817:errorcluster, "NotifyIcon out"=w813:refnum<class "NotifyIcon.lvclass">)  [unwired: 6 in]
  }
  n558 = Index Array(array=w1) -> (element=w54:string)  [unwired: 1 in]
  n559 = property class="NotifyIcon"(reference=w70, error in=w71, "Public:Visible"=TRUE ("Visible"), "Public:DefaultMenuItem"=w54, "Public:TipText"="平台数据传输系统" ("TipText")) -> (reference out=w67:refnum<class "NotifyIcon.lvclass">, error out=w58:errorcluster, "Public:SelectedItemEvent"=w57:refnum<user-event>)
  n560 = register-events(error in=w58, w57) -> (reference out=w28:refnum<event-registration>, error out=w29:errorcluster)  [unwired: 1 in]
  n561 = while {
    shift-right: [w822] -> w65
    shift-left: w29 -> [w821]
    shift-right: [w823] -> w62
    shift-left: w67 -> [w824]
    shift-right: [w820] -> w63
    shift-left: w28 -> [w825]
    tunnel: [w819] -> _
    stop <- w819 stop-if-true
    n562 = case shown="无错误" w821 {
      selector: w821 -> [w827 w862]
      tunnel: w825 -> [w832 w857]
      tunnel: w824 -> [w831 w858]
      tunnel: [w830 w858] -> w823
      tunnel: [w829 w860] -> w822
      tunnel: [w828 FALSE ("Discard?")] -> w819
      tunnel: [w826 w857] -> w820
      frame No Error {
        n563 = event shown="[0] <Public:SelectedItemEvent>: 用户事件" {
          selector: w832 -> [_ _ _]
          dyn-events: [_ _ _] -> w826
          timeout: _ -> [_ _ _]
          tunnel: w827 -> [w835 w846 w855]
          tunnel: [w835 w846 w854] -> w829
          tunnel: [w834 TRUE FALSE ("Discard?")] -> w828
          tunnel: w831 -> [w833 w844 w856]
          tunnel: [w833 w844 w853] -> w830
          event User Event {
            # "5."
            n564 = event-data() -> ("ItemTag"=w836:string)  [unwired: 1 in]
            n565 = case shown="默认" w836 {
              tunnel: [FALSE TRUE] -> w834
              frame Default {
                n566 = Current VI's Path() -> (path=w838:path)
                n567 = Open VI Reference(vi path=w838) -> (vi reference=w839:refnum<vi>)  [unwired: 5 in, 1 out]
                n568 = invoke class="VI" method="FP.Open"(reference=w839, "Activate"=TRUE ("激活？"), "State"=T16."Standard" ("状态")) -> ()  [unwired: 2 in, 5 out]
              }
              frame "EXIT" {
              }
            }
          }
          event "停止输入": Value Change {
            # "5."
            n569 = event-data() -> ()  [unwired: 1 in, 6 out]
            n570 = Stop(stop? (T)=TRUE ("可见")) -> ()
          }
          event Panel Close? {
            # "4."
            n571 = event-data() -> ("VIRef"=w849:refnum<vi>)  [unwired: 1 in, 3 out]
            n572 = invoke class="VI" method="FP.Open"(reference=w849, "State"=T16."Hidden" ("状态")) -> ()  [unwired: 3 in, 5 out]
            n573 = call <vilib>:"ShowBalloonTip.vi"("Balloon Icon"=BalloonIcon."Information", "error in"=w855, "Text"="欢迎使用平台数据传输系统", "NotifyIcon in"=w856) -> ("error out"=w854:errorcluster, "NotifyIcon out"=w853:refnum<class "NotifyIcon.lvclass">)  [unwired: 6 in]
            n574 = event-data("Discard?"=TRUE ("放弃？")) -> ()  [unwired: 1 in, 1 out]
          }
        }
      }
      frame Error {
        n575 = call <vilib>:"Simple Error Handler.vi"("error in (no error)"=w862) -> ("error out"=w861:errorcluster)  [unwired: 4 in, 4 out]
        n576 = call <vilib>:"Clear Errors.vi"("error in (no error)"=w861) -> ("error out"=w860:errorcluster)  [unwired: 5 in, 1 out]
      }
    }
  }
  n577 = Unregister For Events(event registration refnum=w63, error in=w65) -> (error out=w66:errorcluster)
  n578 = call <vilib>:"Destructor.vi"("error in"=w66, "NotifyIcon"=w62) -> ("error out"=w61:errorcluster)  [unwired: 9 in]
  n579 = call <vilib>:"Simple Error Handler.vi"("error in (no error)"=w61) -> ("error out"=→"错误输出":errorcluster)  [unwired: 4 in, 4 out]
  n580 = case shown="\"Run Time System\"" w46 {
    tunnel: w61 -> [_ _ _ _ _ _ _]
    frame "invalid app kind", Default {
    }
    frame "Development System" {
      n581 = Stop(stop? (T)=TRUE ("可见")) -> ()
    }
    frame "Run Time System" {
      n582 = Quit LabVIEW(quit? (T)=TRUE ("退出？(T)")) -> ()
    }
    frame "Student Edition" {
    }
    frame "Embedded LabVIEW" {
    }
    frame "Evaluation" {
    }
    frame "Custom" {
    }
  }
